vi "FPGA_Target_USB_7855R.vi"() -> ()   [LabVIEW 2023]
uses:
  <vilib>/eio/EIONode/EIONode.xnode
  <vilib>/rvi/eio/common/nirviEmuTemplateMethod_errors.vi
  <vilib>/rvi/DataTransferAndStorage/Container/XNode/niFpgaContainer.xnode
  <vilib>/rvi/interface/RandomDataEmulation/nirviRandomDataFpgaReadWriteTemplate.vi
  Tick Count.vi
  <vilib>/rvi/Memory/Memory_Emulation/nirvimemoryEmulation.vi
  <vilib>/rvi/Memory/Memory_Emulation/nirvimemoryFastEmulation.vi
  <vilib>/Platform/TimedLoop/XDataNode/wakeup.ctl
  <vilib>/Platform/TimedLoop/XDataNode/XDNodeRunTimeDep.lvlib
  <vilib>/Platform/TimedLoop/XDataNode/nitl_modes.ctl
  <vilib>/Platform/TimedLoop/XDataNode/timing_clust.ctl
  <vilib>/Platform/TimedLoop/XDataNode/XDataNode.xnode
  <vilib>/rvi/Arithmetic/AddSubMult/XNode/nirviSatArithmetic.xnode
  <vilib>/eio/EIOPropertyNode/EIOPropertyNode.xnode
  <vilib>/rvi/eio/common/nirviEmuTemplatePropertyGet_errors.vi
  <vilib>/rvi/eio/common/nirviEmuTemplatePropertyGet_noerrors.vi
  <vilib>/rvi/eio/common/nirviEmuTemplatePropertySet_errors.vi
  <vilib>/rvi/eio/common/nirviEmuTemplatePropertySet_noerrors.vi
panel:
  out "DIO0":bool
  out "CurrentMeasuredZ":i16
  out "CurrentMeasuredY":i16
  out "CalCoefAo0":cluster{"LSB Weight":u32, "Offset":i32}
  out "CalCoefAo1":cluster{"LSB Weight":u32, "Offset":i32}
  out "CalCoefAo2":cluster{"LSB Weight":u32, "Offset":i32}
  out "CalCoefAo3":cluster{"LSB Weight":u32, "Offset":i32}
  out "CalCoefAo4":cluster{"LSB Weight":u32, "Offset":i32}
  out "CalCoefAo5":cluster{"LSB Weight":u32, "Offset":i32}
  out "CalCoefAo6":cluster{"LSB Weight":u32, "Offset":i32}
  out "CalCoefAo7":cluster{"LSB Weight":u32, "Offset":i32}
  out "CalConstants Ready":bool
  out "CalCoefAi0":cluster{"LSB Weight":u32, "Offset":i32}
  out "CalCoefAi1":cluster{"LSB Weight":u32, "Offset":i32}
  out "CalCoefAi2":cluster{"LSB Weight":u32, "Offset":i32}
  out "CalCoefAi3":cluster{"LSB Weight":u32, "Offset":i32}
  out "CalCoefAi4":cluster{"LSB Weight":u32, "Offset":i32}
  out "CalCoefAi5":cluster{"LSB Weight":u32, "Offset":i32}
  out "CalCoefAi6":cluster{"LSB Weight":u32, "Offset":i32}
  out "CalCoefAi7":cluster{"LSB Weight":u32, "Offset":i32}
  out "Invert AO4 Output (V2)":bool
  out "Invert AO3 Output (V1)":bool
  out "Move Z Picomotor Direction":bool
  out "Move Z Picomotor":bool
  out "Tick Count(Ticks)":u32
  in  "HoldTimerScale":u64=18446744073709526080
  in  "Feedback1 on  Hold":bool
  out "Feedback2 Error":i32
  out "Feedback1 Error":i32
  out "Feedback2 Boolean":bool
  out "Feedback1 Boolean":bool
  out "ExtraTime 4":fxp<+,64,64>
  in  "DistanceToBulk 3":i16
  in  "DistanceToBulk 2":i16
  out "HasHeldHoldTimeHappend?":bool
  out "Z_axis_-10Vto10V":bool
  out "TraceRetraceFirstUse":bool
  in  "DistanceToBulk":i16
  out "V START":i16
  out "V END":i16
  out "X START":i16
  out "Y START":i16
  out "Z START":i16
  out "X END":i16
  out "Y END":i16
  out "Z END":i16
  out "V2 START":i16
  out "Count Average":i16
  out "AverageSum":i64
  out "IterateHolder":i16
  out "V2 VEl":i16
  out "V2 END":i16
  out "Update Position Loop Wait Time (ms)":u16=1
  out "LineType":i16
  out "V VEl":i16
  out "Z VEL":i16
  out "Y VEL":i16
  out "X VEL":i16
  out "Element":i16
  in  "V on Fly":i16=-32768
  in  "Change V on Fly":bool
  in  "Feedback_Threshold":i32
  in  "FeedBackType":u8
  out "x < y?":bool
  out "ExtraTime 3":fxp<+,64,64>
  in  "P2AvgMinus":i32
  out "ExtraTime 2":fxp<+,64,64>
  in  "P2AvgWhole":i32
  in  "Xoffset":u32
  in  "P":fxp<+/-,32,1>
  in  "Upper limit Of dZ":i32
  in  "FeedBackType 2":u8
  in  "Feedback_Threshold 2":i32
  in  "GreaterThan 2":bool
  in  "GreaterThan":bool
  in  "V2 on Fly":i16=-32768
  in  "Change V on Fly 2":bool
  out "CurrentMeasuredX":i16
  in  "2^(-n)":i16
  out "SampleNum":i16
  in  "Buffer Loop Wait Time (tICKS)":u32=1
  out "SampleIterator":i16
  out "Internal Stop":bool caption="Stop"
  out "MeasuredCurrent":i16=32767
  out "Applied Voltage":i16=-32768
  in  "External Stop":bool caption="Stop"
  in  "External Pause":bool
  out "Applied Z":i16
  out "Applied Y":i16
  out "Applied X":i16
  in  "Internal Pause":bool
  out "Accum Z":i32
  out "Accum I":i32
  out "Accum dV":i32
  out "Accum I2":i32
  out "OnlyStopLineONCE X":bool
  out "Accum Ext ac":i32
  out "Ext amp":i16=32767
  out "Accum Ext phase":i32
  in  "ExpandVelScaller X":i16=-27
  out "LineNumber":u64
  out "WaitingForWayPoints":bool caption="Stop"
  out "HoldTimer (ticks)":u64
  out "MeasuredCurrent 2":i16=32767
  out "Ext Phase":i16=32767
  in  "ExpandVelScaller Y":i16=-27
  in  "ExpandVelScaller Z":i16=-27
  in  "ExpandVelScaller V":i16=-27
  out "Accum I3":i32
  out "MeasuredCurrent 3":i16=32767
  out "MeasuredCurrent 4":i16=32767
  out "Accum Y":i32
  out "Accum X":i32
  out "OnlyStopLineONCE Y":bool
  out "OnlyStopLineONCE Z":bool
  out "OnlyStopLineONCE V":bool
  in  "EndCurrentLine":bool
  out "StopMoveX":bool
  out "StopMoveY":bool
  out "StopMoveZ":bool
  out "StopMoveV":bool
  out "Jump V":bool
  out "Stop Hold Position":bool
  out "Applied Voltage 2":i16
  out "StopMoveV2":bool
  out "Accum dV2":i32
  out "Jump V2":bool
  in  "ExpandVelScaller V2":i16=-27
  out "OnlyStopLineONCE V2":bool
  out "MoveAverage":i16
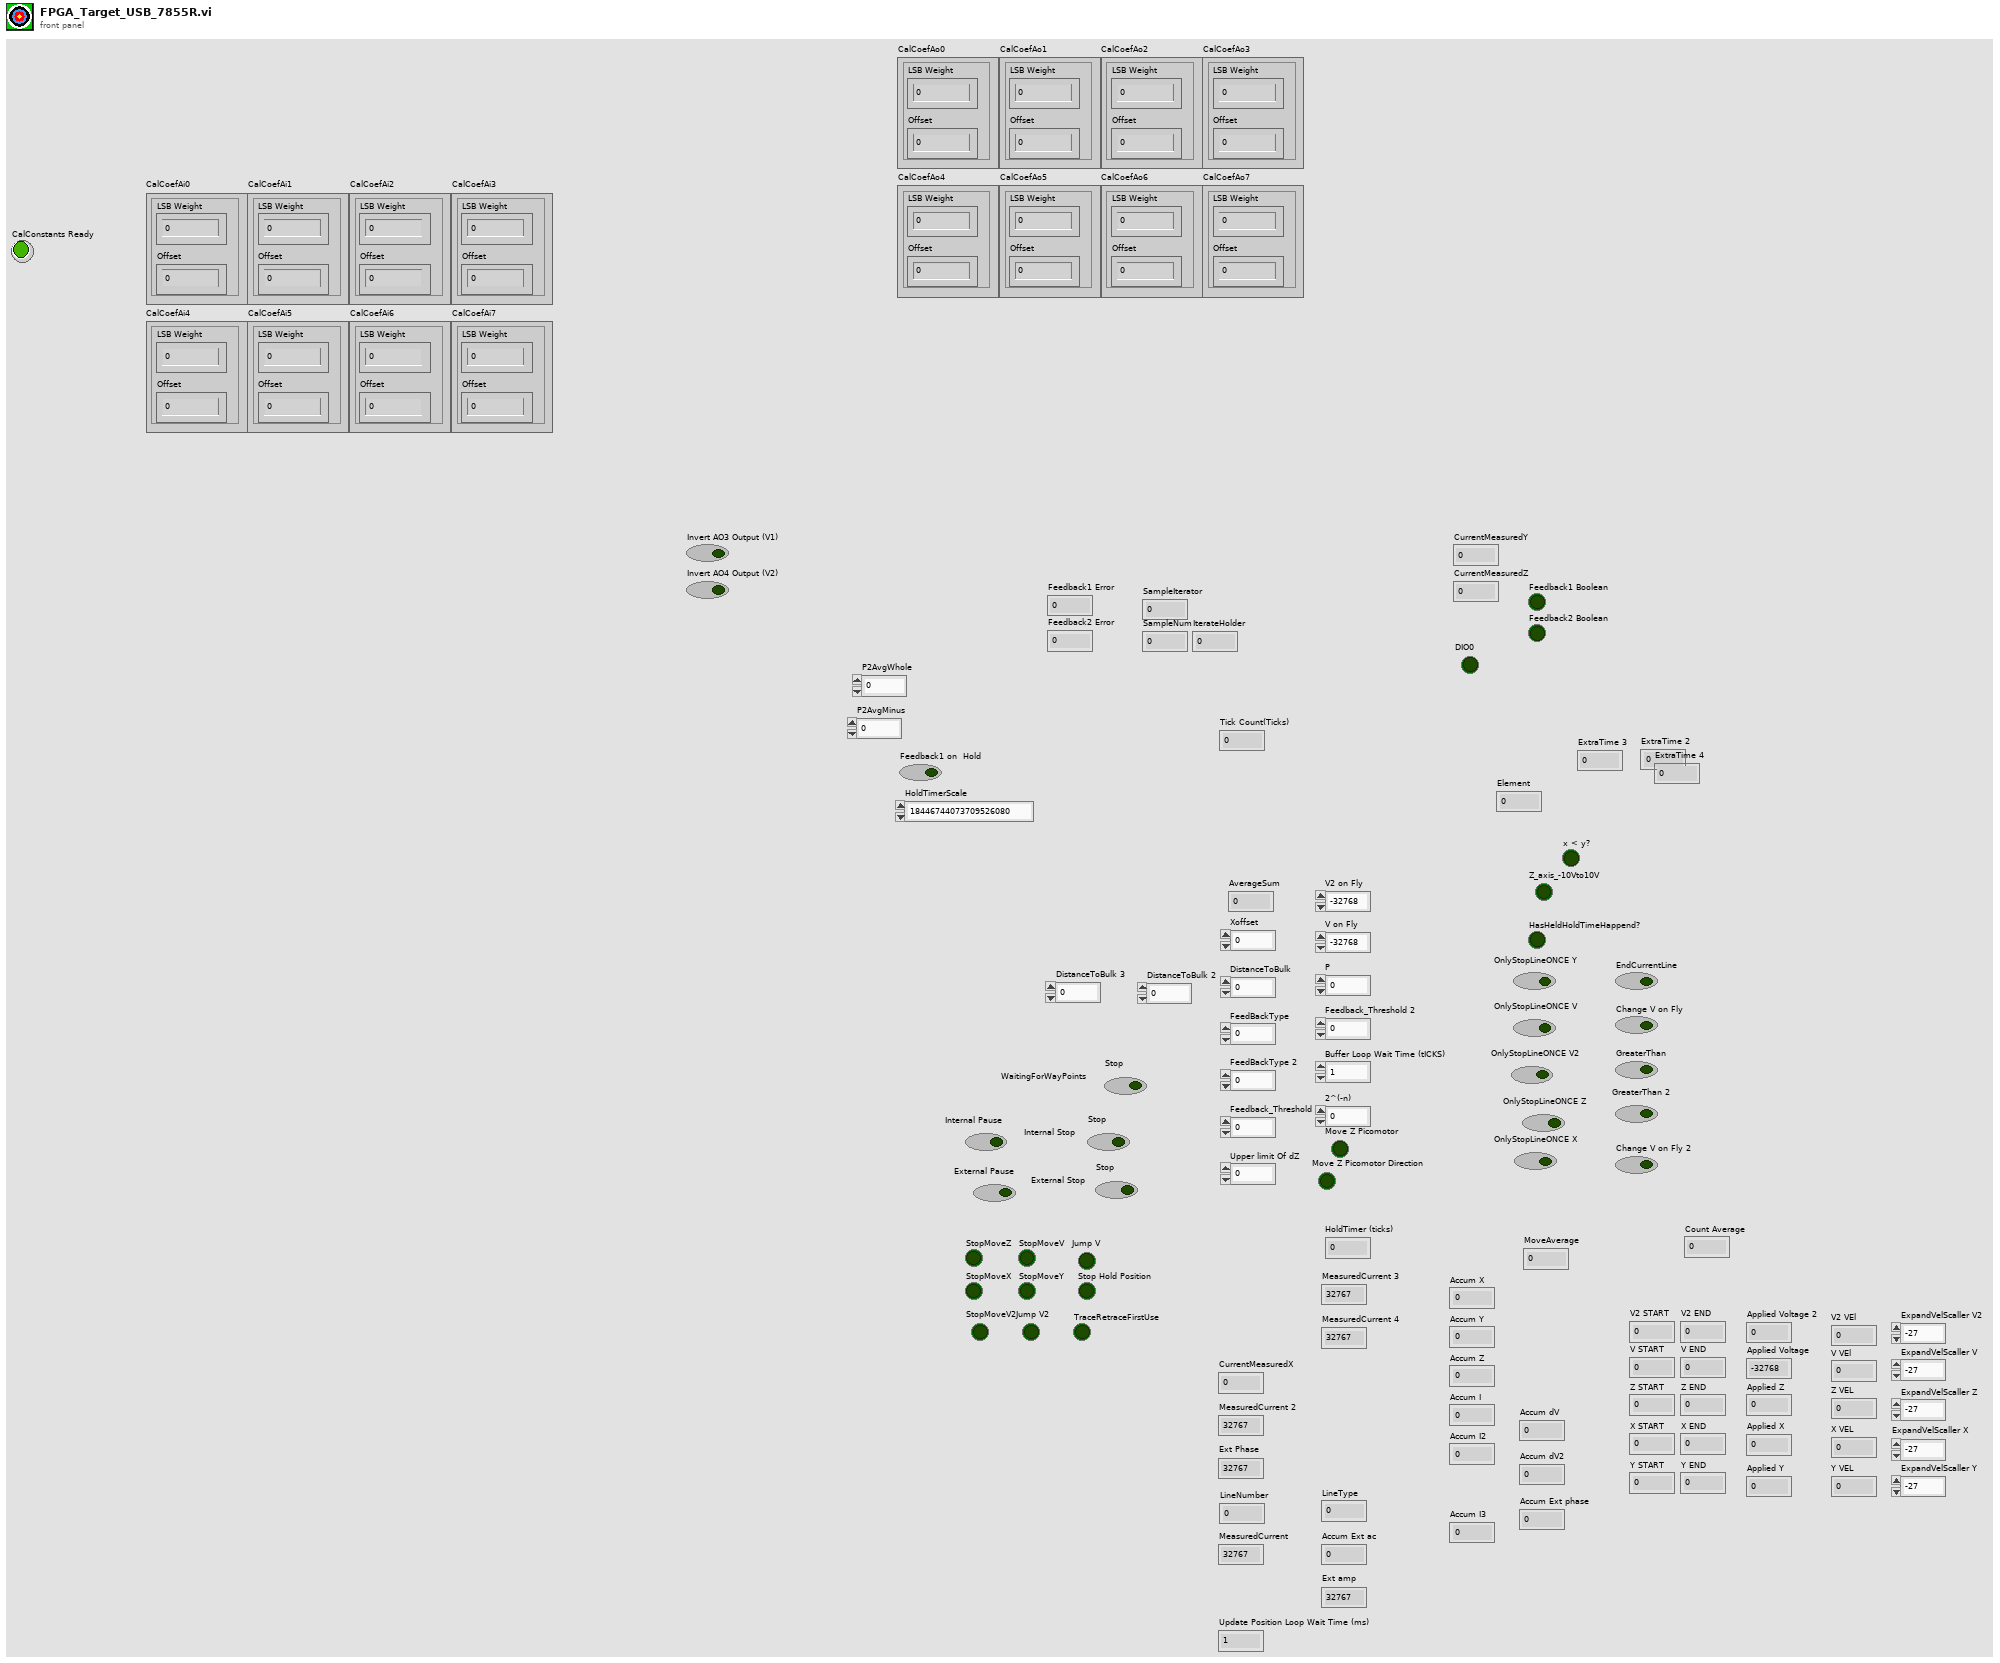
[diagram p1: front panel]
types:
  T1 = typedef "XDNodeRunTimeDep.lvlib/timing_clust.ctl" = cluster{"Expected End [f-1]":u64, "Actual End [f-1]":u64, "Finished Late? [f-1]":bool, "Expected End [i-1]":u64, "Actual End [i-1]":u64, "Finished Late? [i-1]":bool, "Expected Start [i]":u64, "Actual Start [i]":u64, "Expected Start [f]":u64, "Actual Start [f]":u64, "Source Name":string, "Structure Name":string, "Period":i64, "Deadline":i64, "Offset":i64, "Start":i64, "Priority":i32, "Timeout":i32, "Mode":T2, "Wakeup Reason":T3, "Error":errorcluster, "Source Type":string, "Secondary Source Type":string, "Global End Time":u64, "Global Start Time":u64, "Frame Duration":u64, "Iteration Duration":u64, "Assigned CPU":i32, "I/O Scan Engine Mode":u32}
  T2 = typedef "XDNodeRunTimeDep.lvlib/nitl_modes.ctl" = enum32{"No Change", "Process missed periods, maintain original phase", "Discard missed periods, maintain original phase", "Process missed periods, ignore original phase", "Discard missed periods, ignore original phase"}
  T3 = typedef "XDNodeRunTimeDep.lvlib/wakeup.ctl" = enum32{"Normal", "Aborted", "Asynchronous wakeup", "Timing source error", "Timed loop error", "Timeout"}
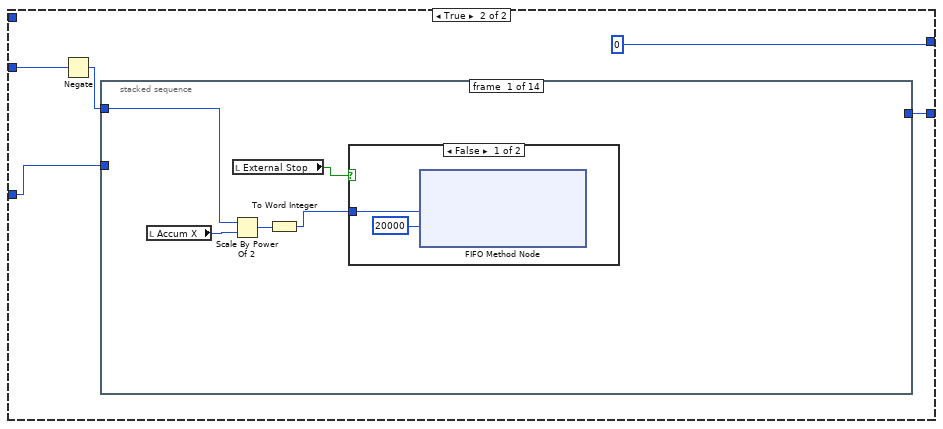
[diagram p2: hidden frame]
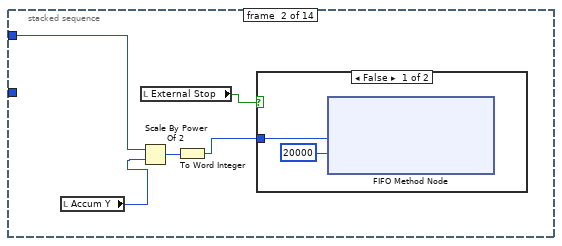
[diagram p4: hidden frame]
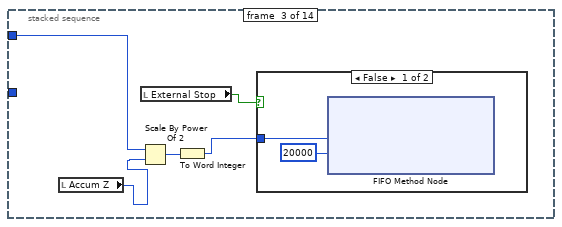
[diagram p6: hidden frame]
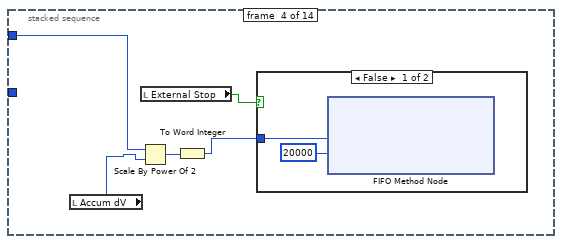
[diagram p8: hidden frame]
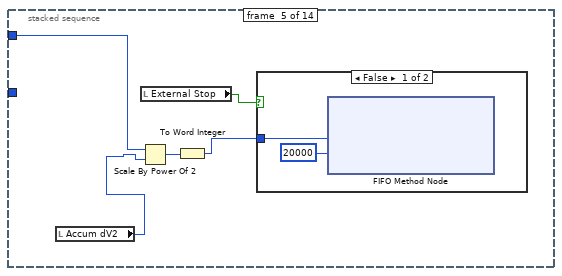
[diagram p10: hidden frame]
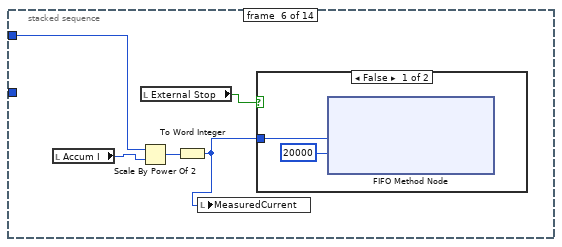
[diagram p12: hidden frame]
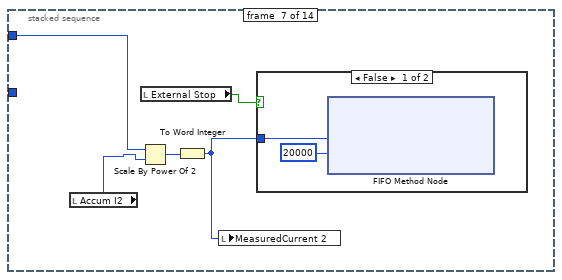
[diagram p14: hidden frame]
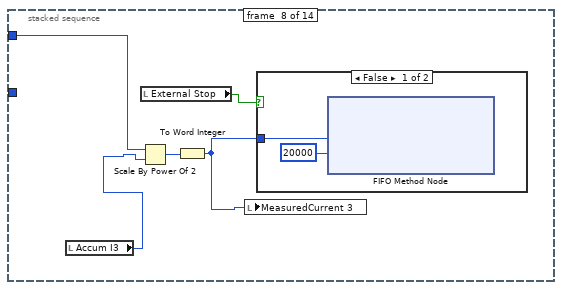
[diagram p16: hidden frame]
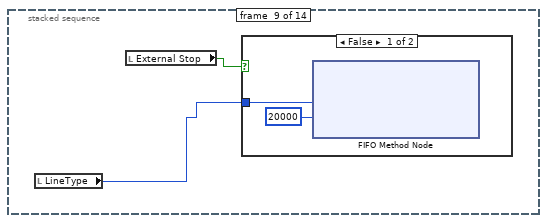
[diagram p18: hidden frame]
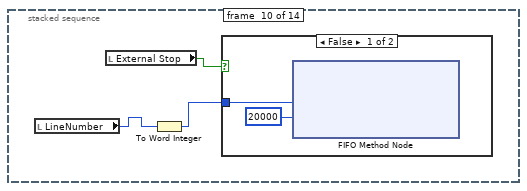
[diagram p20: hidden frame]
diagram:
  # "Increments  tick count by one every cycle, looping back to zero at ~2e19 ticks"
  n1 = node-c288() -> (w3:T1)  [unwired: 1 in]
  n2 = flat-sequence {
    frame #0 {
      w5 = FALSE ("Invert AO4 Output (V2)")
      w10 = FALSE ("OnlyStopLineONCE V2")
      w11 = FALSE ("Internal Stop")
      w4 = FALSE ("Internal Stop")
      w8 = u64 0 ("LineNumber")
      w7 = i16 0 ("Ext amp")
      w9 = i16 0 ("Applied Volatge")
      w18 = i16 32767 ("dZ Position")
      # "Set initial values of FP items and voltages to AO channels"
      "Internal Stop" <- FALSE ("Internal Stop")
      "MeasuredCurrent" <- w18
      "Applied Voltage" <- w9
      "Applied Z" <- i16 16383 ("Applied Volatge")
      "Applied Y" <- i16 16383 ("Applied Volatge")
      "Applied X" <- i16 16383 ("Applied Volatge")
      "Accum Z" <- 0 ("Applied Volatge")
      "Accum I" <- 0 ("Applied Volatge")
      "Accum dV" <- 0 ("Applied Volatge")
      "Accum I2" <- 0 ("Applied Volatge")
      "OnlyStopLineONCE X" <- w10
      "Accum Ext ac" <- 0 ("Accum Ext ac")
      "Ext amp" <- w7
      "Accum Ext phase" <- 0 ("Accum Ext phase")
      "LineNumber" <- w8
      "WaitingForWayPoints" <- FALSE ("WaitingForWayPoints")
      "HoldTimer (ticks)" <- w8
      "MeasuredCurrent 2" <- w18
      "Ext Phase" <- w7
      "Accum I3" <- 0 ("Applied Volatge")
      "MeasuredCurrent 3" <- w18
      "MeasuredCurrent 4" <- w18
      "Accum Y" <- 0 ("Applied Volatge")
      "Accum X" <- 0 ("Applied Volatge")
      "OnlyStopLineONCE Y" <- w10
      "OnlyStopLineONCE Z" <- w10
      "OnlyStopLineONCE V" <- w10
      "StopMoveX" <- w11
      "StopMoveY" <- w11
      "StopMoveZ" <- w11
      "StopMoveV" <- w11
      "Jump V" <- w4
      "Stop Hold Position" <- w4
      "Applied Voltage 2" <- w9
      "StopMoveV2" <- w11
      "Accum dV2" <- 0 ("Applied Volatge")
      "Jump V2" <- w4
      "OnlyStopLineONCE V2" <- w10
      "MoveAverage" <- w7
      "Z_axis_-10Vto10V" <- FALSE ("Internal Stop")
      "Move Z Picomotor" <- w4
      "Move Z Picomotor Direction" <- w4
      "Invert AO3 Output (V1)" <- w5
      "Invert AO4 Output (V2)" <- w5
      "DIO0" <- w4
    }
    frame #1 {
      w29 = i16 0  # SampleIterator
      n3 = while "Data Collection and Buffering Loop" {
        shift-right: [w34] -> _
        shift-left: w29 -> [w35]
        shift-right: [w32] -> _
        shift-left: u32 0 ("Tick Count(Ticks)") -> [w30]
        stop <- FALSE stop-if-true
        n4 = flat-sequence {
          tunnel: [w39] -> w36
          tunnel: w35 -> [w39]
          tunnel: w30 -> [w37]
          tunnel: [w37] -> w31
          tunnel: w36 -> [w47]
          tunnel: [w46] -> w34
          tunnel: [w41] -> w32
          tunnel: w31 -> [w40]
          frame #0 {
            n5 = call "Loop Timer2"("Count(Ticks)"="Buffer Loop Wait Time (tICKS)") -> ()  [unwired: 1 out]
          }
          frame #1 {
            n6 = Scale By Power Of 2(n="2^(-n)", x=i16 1) -> (x*2^n=w44:i16)
            "SampleNum" <- w44
            n7 = Greater Or Equal?(x=w47, y=w44) -> (x >= y?=w42:bool)
            n8 = case shown="False" w42 {
              tunnel: w47 -> [w90 _]
              tunnel: [w89 i16 0 ("lo")] -> w46
              tunnel: "2^(-n)" -> [_ w94]
              tunnel: [w48 w92] -> w41
              tunnel: w40 -> [w48 w91]
              frame False {
                n9 = xnode "FPGA I/O Node"() -> ("Connector1/AI0"=w53, "Connector1/AI1"=w60, "Connector1/AI2"=w77, "Connector1/AI3"=w76, "Connector1/AI4"=w75, "Connector1/AI5"=w74, "Connector1/AI6"=w67, "Connector1/AI7"=w64)  [unwired: 8 in, 8 out]
                "CurrentMeasuredX" <- w53
                "CurrentMeasuredY" <- w60
                "CurrentMeasuredZ" <- w77
                n10 = local read "Applied Voltage 2"() -> (w51:i16)
                n11 = local read "Applied Voltage"() -> (w79:i16)
                n12 = Increment(x=w90) -> (x+1=w89:i16)
                n13 = To Long Integer(number=w79) -> (32bit integer=w78:i32)
                n14 = To Long Integer(number=w51) -> (32bit integer=w52:i32)
                n15 = To Long Integer(number=w64) -> (32bit integer=w63:i32)
                n16 = To Long Integer(number=w77) -> (32bit integer=w61:i32)
                n17 = To Long Integer(number=w53) -> (32bit integer=w54:i32)
                n18 = To Long Integer(number=w60) -> (32bit integer=w59:i32)
                n19 = To Long Integer(number=w74) -> (32bit integer=w73:i32)
                n20 = local read "Accum dV2"() -> (w49:i32)
                n21 = local read "Accum dV"() -> (w81:i32)
                n22 = To Long Integer(number=w75) -> (32bit integer=w83:i32)
                n23 = local read "Accum I3"() -> (w65:i32)
                n24 = To Long Integer(number=w76) -> (32bit integer=w86:i32)
                n25 = local read "Accum X"() -> (w55:i32)
                n26 = local read "Accum Ext phase"() -> (w69:i32)
                n27 = local read "Accum Y"() -> (w58:i32)
                n28 = local read "Accum I2"() -> (w84:i32)
                n29 = local read "Accum Ext ac"() -> (w72:i32)
                n30 = local read "Accum Z"() -> (w62:i32)
                n31 = local read "Accum I"() -> (w87:i32)
                n32 = Add(x=w81, y=w78) -> (x+y=w80:i32)
                n33 = Add(x=w49, y=w52) -> (x+y=w50:i32)
                n34 = To Long Integer(number=w67) -> (32bit integer=w68:i32)
                n35 = Add(x=w55, y=w54) -> (x+y=w56:i32)
                n36 = Add(x=w58, y=w59) -> (x+y=w57:i32)
                n37 = Add(x=w62, y=w61) -> (x+y=w88:i32)
                n38 = Add(x=w84, y=w83) -> (x+y=w82:i32)
                n39 = Add(x=w63, y=w65) -> (x+y=w66:i32)
                n40 = Add(x=w87, y=w86) -> (x+y=w85:i32)
                n41 = Add(x=w68, y=w69) -> (x+y=w70:i32)
                n42 = Add(x=w72, y=w73) -> (x+y=w71:i32)
                n43 = local write "Accum dV2"(w50) -> ()
                n44 = local write "Accum dV"(w80) -> ()
                n45 = local write "Accum X"(w56) -> ()
                n46 = local write "Accum Ext phase"(w70) -> ()
                n47 = local write "Accum Y"(w57) -> ()
                n48 = local write "Accum Ext ac"(w71) -> ()
                n49 = local write "Accum Z"(w88) -> ()
                n50 = local write "Accum I2"(w82) -> ()
                n51 = local write "Accum I"(w85) -> ()
                n52 = local write "Accum I3"(w66) -> ()
              }
              frame True {
                n53 = Negate(x=w94) -> (-x=w93:i16)
                n54 = stacked-sequence {
                  tunnel: w93 -> [w96 w104 w111 w119 w126 w133 w140 w147 _ _ w164 w171 _ _]
                  tunnel: [_ _ _ _ _ _ _ _ _ _ _ _ w177 _] -> w92
                  tunnel: w91 -> [_ _ _ _ _ _ _ _ _ _ _ _ w176 _]
                  frame #0 {
                    n55 = local read "Accum X"() -> (w97:i32)
                    n56 = Scale By Power Of 2(n=w96, x=w97) -> (x*2^n=w98:i32)
                    n57 = local read "External Stop"() -> (w99:bool)
                    n58 = To Word Integer(number=w98) -> (16bit integer=w100:i16)
                    n59 = case shown="False" w99 {
                      tunnel: w100 -> [w101 _]
                      frame False {
                        n60 = xnode ("FIFO Method Node")("Element"=w101, "Timeout"=20000) -> ()  [unwired: 1 in, 2 out]
                      }
                      frame True {
                      }
                    }
                  }
                  frame #1 {
                    n61 = local read "Accum Y"() -> (w103:i32)
                    n62 = Scale By Power Of 2(n=w104, x=w103) -> (x*2^n=w105:i32)
                    n63 = local read "External Stop"() -> (w106:bool)
                    n64 = To Word Integer(number=w105) -> (16bit integer=w107:i16)
                    n65 = case shown="False" w106 {
                      tunnel: w107 -> [w108 _]
                      frame False {
                        n66 = xnode ("FIFO Method Node")("Element"=w108, "Timeout"=20000) -> ()  [unwired: 1 in, 2 out]
                      }
                      frame True {
                      }
                    }
                  }
                  frame #2 {
                    n67 = local read "Accum Z"() -> (w110:i32)
                    n68 = Scale By Power Of 2(n=w111, x=w110) -> (x*2^n=w112:i32)
                    n69 = local read "External Stop"() -> (w113:bool)
                    n70 = To Word Integer(number=w112) -> (16bit integer=w114:i16)
                    n71 = case shown="False" w113 {
                      tunnel: w114 -> [w115 _]
                      frame False {
                        n72 = xnode ("FIFO Method Node")("Element"=w115, "Timeout"=20000) -> ()  [unwired: 1 in, 2 out]
                      }
                      frame True {
                      }
                    }
                  }
                  frame #3 {
                    n73 = local read "Accum dV"() -> (w117:i32)
                    n74 = Scale By Power Of 2(n=w119, x=w117) -> (x*2^n=w120:i32)
                    n75 = local read "External Stop"() -> (w121:bool)
                    n76 = To Word Integer(number=w120) -> (16bit integer=w118:i16)
                    n77 = case shown="False" w121 {
                      tunnel: w118 -> [w122 _]
                      frame False {
                        n78 = xnode ("FIFO Method Node")("Element"=w122, "Timeout"=20000) -> ()  [unwired: 1 in, 2 out]
                      }
                      frame True {
                      }
                    }
                  }
                  frame #4 {
                    n79 = local read "Accum dV2"() -> (w124:i32)
                    n80 = Scale By Power Of 2(n=w126, x=w124) -> (x*2^n=w127:i32)
                    n81 = local read "External Stop"() -> (w128:bool)
                    n82 = To Word Integer(number=w127) -> (16bit integer=w125:i16)
                    n83 = case shown="False" w128 {
                      tunnel: w125 -> [w129 _]
                      frame False {
                        n84 = xnode ("FIFO Method Node")("Element"=w129, "Timeout"=20000) -> ()  [unwired: 1 in, 2 out]
                      }
                      frame True {
                      }
                    }
                  }
                  frame #5 {
                    n85 = local read "Accum I"() -> (w132:i32)
                    n86 = Scale By Power Of 2(n=w133, x=w132) -> (x*2^n=w134:i32)
                    n87 = local read "External Stop"() -> (w135:bool)
                    n88 = To Word Integer(number=w134) -> (16bit integer=w131:i16)
                    n89 = local write "MeasuredCurrent"(w131) -> ()
                    n90 = case shown="False" w135 {
                      tunnel: w131 -> [w136 _]
                      frame False {
                        n91 = xnode ("FIFO Method Node")("Element"=w136, "Timeout"=20000) -> ()  [unwired: 1 in, 2 out]
                      }
                      frame True {
                      }
                    }
                  }
                  frame #6 {
                    n92 = local read "Accum I2"() -> (w139:i32)
                    n93 = Scale By Power Of 2(n=w140, x=w139) -> (x*2^n=w141:i32)
                    n94 = local read "External Stop"() -> (w142:bool)
                    n95 = To Word Integer(number=w141) -> (16bit integer=w138:i16)
                    n96 = local write "MeasuredCurrent 2"(w138) -> ()
                    n97 = case shown="False" w142 {
                      tunnel: w138 -> [w143 _]
                      frame False {
                        n98 = xnode ("FIFO Method Node")("Element"=w143, "Timeout"=20000) -> ()  [unwired: 1 in, 2 out]
                      }
                      frame True {
                      }
                    }
                  }
                  frame #7 {
                    n99 = local read "Accum I3"() -> (w146:i32)
                    n100 = Scale By Power Of 2(n=w147, x=w146) -> (x*2^n=w148:i32)
                    n101 = local read "External Stop"() -> (w149:bool)
                    n102 = To Word Integer(number=w148) -> (16bit integer=w145:i16)
                    n103 = local write "MeasuredCurrent 3"(w145) -> ()
                    n104 = case shown="False" w149 {
                      tunnel: w145 -> [w150 _]
                      frame False {
                        n105 = xnode ("FIFO Method Node")("Element"=w150, "Timeout"=20000) -> ()  [unwired: 1 in, 2 out]
                      }
                      frame True {
                      }
                    }
                  }
                  frame #8 {
                    n106 = local read "LineType"() -> (w152:i16)
                    n107 = local read "External Stop"() -> (w153:bool)
                    n108 = case shown="False" w153 {
                      tunnel: w152 -> [w154 _]
                      frame False {
                        n109 = xnode ("FIFO Method Node")("Element"=w154, "Timeout"=20000) -> ()  [unwired: 1 in, 2 out]
                      }
                      frame True {
                      }
                    }
                  }
                  frame #9 {
                    n110 = local read "LineNumber"() -> (w157:u64)
                    n111 = local read "External Stop"() -> (w158:bool)
                    n112 = To Word Integer(number=w157) -> (16bit integer=w156:i16)
                    n113 = case shown="False" w158 {
                      tunnel: w156 -> [w159 _]
                      frame False {
                        n114 = xnode ("FIFO Method Node")("Element"=w159, "Timeout"=20000) -> ()  [unwired: 1 in, 2 out]
                      }
                      frame True {
                      }
                    }
                  }
                  frame #10 {
                    n115 = local read "Accum Ext ac"() -> (w163:i32)
                    n116 = local read "External Stop"() -> (w165:bool)
                    n117 = Scale By Power Of 2(n=w164, x=w163) -> (x*2^n=w162:i32)
                    n118 = To Word Integer(number=w162) -> (16bit integer=w161:i16)
                    n119 = case shown="False" w165 {
                      tunnel: w161 -> [w166 _]
                      frame False {
                        n120 = xnode ("FIFO Method Node")("Element"=w166, "Timeout"=20000) -> ()  [unwired: 1 in, 2 out]
                      }
                      frame True {
                      }
                    }
                    n121 = local write "Ext amp"(w161) -> ()
                  }
                  frame #11 {
                    n122 = local read "Accum Ext phase"() -> (w169:i32)
                    n123 = local read "External Stop"() -> (w172:bool)
                    n124 = Scale By Power Of 2(n=w171, x=w169) -> (x*2^n=w170:i32)
                    n125 = To Word Integer(number=w170) -> (16bit integer=w168:i16)
                    n126 = local write "Ext Phase"(w168) -> ()
                    n127 = case shown="False" w172 {
                      tunnel: w168 -> [w173 _]
                      frame False {
                        n128 = xnode ("FIFO Method Node")("Element"=w173, "Timeout"=20000) -> ()  [unwired: 1 in, 2 out]
                      }
                      frame True {
                      }
                    }
                  }
                  frame #12 {
                    n129 = call "Tick Count"() -> ("Tick Count(Ticks)"=w177:u32)
                    n130 = Subtract(x=w177, y=w176) -> (x-y=w175:u32)
                    "Tick Count(Ticks)" <- w175
                    n131 = local read "External Stop"() -> (w188:bool)
                    n132 = Split Number(x=w175) -> (hi(x)=w187:u16, lo(x)=w179:u16)
                    n133 = To Long Integer(number=w179) -> (32bit integer=w180:i32)
                    n134 = To Long Integer(number=w187) -> (32bit integer=w186:i32)
                    n135 = Subtract(x=w180, y=32768) -> (x-y=w182:i32)
                    n136 = Subtract(x=w186, y=32768) -> (x-y=w184:i32)
                    n137 = To Word Integer(number=w182) -> (16bit integer=w178:i16)
                    n138 = To Word Integer(number=w184) -> (16bit integer=w183:i16)
                    n139 = case shown="False" w188 {
                      tunnel: w183 -> [w190 _]
                      tunnel: w178 -> [w189 _]
                      frame False {
                        n140 = flat-sequence {
                          tunnel: w190 -> [w191]
                          tunnel: w189 -> [w193]
                          frame #0 {
                            n141 = xnode ("FIFO Method Node")("Element"=w191, "Timeout"=20000) -> ()  [unwired: 1 in, 2 out]
                          }
                          frame #1 {
                            n142 = xnode ("FIFO Method Node")("Element"=w193, "Timeout"=20000) -> ()  [unwired: 1 in, 2 out]
                          }
                        }
                      }
                      frame True {
                      }
                    }
                  }
                  frame #13 {
                    n143 = local write "Accum dV"(0 ("MeasuredCurrent")) -> ()
                    n144 = local write "Accum Z"(0 ("MeasuredCurrent")) -> ()
                    n145 = local write "Accum dV2"(0 ("Accum Ext ac")) -> ()
                    n146 = local write "Accum I2"(0 ("MeasuredCurrent")) -> ()
                    n147 = local write "Accum I"(0 ("MeasuredCurrent")) -> ()
                    n148 = local write "Accum Y"(0 ("Accum Ext ac")) -> ()
                    n149 = local write "Accum X"(0 ("MeasuredCurrent")) -> ()
                    n150 = local write "Accum Ext ac"(0 ("Accum Ext ac")) -> ()
                    n151 = local write "Accum I3"(0 ("Accum Ext ac")) -> ()
                    n152 = local write "Accum Ext phase"(0 ("Accum Ext phase")) -> ()
                  }
                }
              }
            }
          }
        }
        "SampleIterator" <- w35
      }
      n153 = while "X Y Z Voltage" {
        stop <- FALSE stop-if-true
        # "Load Waypoints"
        n154 = flat-sequence {
          tunnel: [w1129] -> w206
          tunnel: [w1128] -> w212
          tunnel: [w1127] -> w211
          tunnel: [w1126] -> w210
          tunnel: [w1125] -> w209
          tunnel: [w1124] -> w208
          tunnel: [w1122] -> w207
          tunnel: [w1121] -> w205
          frame #0 {
            n155 = while {
              shift-right: [w922] -> _
              shift-left: TRUE ("WaitingForWayPoints") -> [w923]
              stop <- w926 stop-if-true
              n156 = xnode ("FIFO Method Node")() -> ("Number of Elements to Read"=w931:u32)  [unwired: 1 in, 1 out]
              n157 = local read "External Stop"() -> (w924:bool)
              n158 = And(x=w924, y=w923) -> (x .and. y?=w925:bool)
              n159 = case shown="True" w925 {
                tunnel: w923 -> [w932 _]
                tunnel: [w932 FALSE ("WaitingForWayPoints")] -> w922
                frame False {
                }
                frame True {
                  n160 = while {
                    stop <- w934 stop-if-true
                    n161 = xnode ("FIFO Method Node")("Timeout"=100) -> ("Element"=→"Element":i16, "Timed Out?"=w934:bool)  [unwired: 1 in, 1 out]
                  }
                }
              }
              n162 = Greater?(x=w931, y=u32 13) -> (0:w927:bool)
              n163 = Not(x=w927) -> (.not. x?=w929:bool)
              n164 = local write "WaitingForWayPoints"(w929) -> ()
              n165 = Not(x=w924) -> (.not. x?=w928:bool)
              n166 = And(x=w928, y=w927) -> (x .and. y?=w926:bool)
            }
          }
          frame #1 {
            n167 = stacked-sequence {
              frame #0 {
                n168 = xnode ("FIFO Method Node")("Timeout"=-1) -> ("Element"=→"LineType":i16)  [unwired: 1 in, 2 out]
              }
              frame #1 {
                n169 = xnode ("FIFO Method Node")("Timeout"=-1) -> ("Element"=→"X VEL":i16)  [unwired: 1 in, 2 out]
              }
              frame #2 {
                n170 = xnode ("FIFO Method Node")("Timeout"=-1) -> ("Element"=→"Y VEL":i16)  [unwired: 1 in, 2 out]
              }
              frame #3 {
                n171 = xnode ("FIFO Method Node")("Timeout"=-1) -> ("Element"=→"Z VEL":i16)  [unwired: 1 in, 2 out]
              }
              frame #4 {
                n172 = xnode ("FIFO Method Node")("Timeout"=-1) -> ("Element"=→"V VEl":i16)  [unwired: 1 in, 2 out]
              }
              frame #5 {
                n173 = xnode ("FIFO Method Node")("Timeout"=-1) -> ("Element"=→"V2 VEl":i16)  [unwired: 1 in, 2 out]
              }
              frame #6 {
                n174 = xnode ("FIFO Method Node")("Timeout"=-1) -> ("Element"=→"X END":i16)  [unwired: 1 in, 2 out]
              }
              frame #7 {
                n175 = xnode ("FIFO Method Node")("Timeout"=-1) -> ("Element"=→"Y END":i16)  [unwired: 1 in, 2 out]
              }
              frame #8 {
                n176 = xnode ("FIFO Method Node")("Timeout"=-1) -> ("Element"=w954:i16)  [unwired: 1 in, 2 out]
                n177 = local read "LineType"() -> (w955:i16)
                n178 = case shown="13" w955 {
                  tunnel: [w957 w962 w974 w986 w994] -> w953
                  tunnel: w954 -> [w957 _ _ _ _]
                  frame 0..2, Default {
                    # "Normal Move"
                  }
                  frame 3 {
                    # "Bulk At End Of line - Retract"
                    n179 = local read "Z_axis_-10Vto10V"() -> (w961:bool)
                    n180 = local read "Applied Z"() -> (w969:i16)
                    n181 = Select(t=-32768 ("lower limit"), s=w961, f=0 ("lower limit")) -> (s? t:f=w960:i32)
                    n182 = To Long Integer(number=w969) -> (32bit integer=w966:i32)
                    n183 = To Long Integer(number="DistanceToBulk") -> (32bit integer=w967:i32)
                    n184 = Add(x=w966, y=w967) -> (x+y=w965:i32)
                    n185 = In Range and Coerce(upper limit=32767, x=w965, lower limit=w960) -> (coerced(x)=w963:i32)  [unwired: 1 out]
                    n186 = To Word Integer(number=w963) -> (16bit integer=w962:i16)
                  }
                  frame 12 {
                    # "Bulk At End Of line - Retract"
                    n187 = local read "Z_axis_-10Vto10V"() -> (w973:bool)
                    n188 = local read "Applied Z"() -> (w981:i16)
                    n189 = Select(t=-32768 ("lower limit"), s=w973, f=0 ("lower limit")) -> (s? t:f=w972:i32)
                    n190 = To Long Integer(number=w981) -> (32bit integer=w978:i32)
                    n191 = To Long Integer(number="DistanceToBulk 2") -> (32bit integer=w979:i32)
                    n192 = Add(x=w978, y=w979) -> (x+y=w977:i32)
                    n193 = In Range and Coerce(upper limit=32767, x=w977, lower limit=w972) -> (coerced(x)=w975:i32)  [unwired: 1 out]
                    n194 = To Word Integer(number=w975) -> (16bit integer=w974:i16)
                  }
                  frame 13 {
                    # "Bulk At End Of line - Retract"
                    n195 = local read "Z_axis_-10Vto10V"() -> (w985:bool)
                    n196 = local read "Applied Z"() -> (w993:i16)
                    n197 = Select(t=-32768 ("lower limit"), s=w985, f=0 ("lower limit")) -> (s? t:f=w984:i32)
                    n198 = To Long Integer(number=w993) -> (32bit integer=w990:i32)
                    n199 = To Long Integer(number="DistanceToBulk 3") -> (32bit integer=w991:i32)
                    n200 = Add(x=w990, y=w991) -> (x+y=w989:i32)
                    n201 = In Range and Coerce(upper limit=32767, x=w989, lower limit=w984) -> (coerced(x)=w987:i32)  [unwired: 1 out]
                    n202 = To Word Integer(number=w987) -> (16bit integer=w986:i16)
                  }
                  frame 4..7 {
                    # "Start at current hieght"
                    n203 = local read "Applied Z"() -> (w994:i16)
                  }
                }
                "Z END" <- w953
              }
              frame #9 {
                n204 = xnode ("FIFO Method Node")("Timeout"=-1) -> ("Element"=→"V END":i16)  [unwired: 1 in, 2 out]
              }
              frame #10 {
                n205 = xnode ("FIFO Method Node")("Timeout"=-1) -> ("Element"=→"V2 END":i16)  [unwired: 1 in, 2 out]
              }
              frame #11 {
                n206 = xnode ("FIFO Method Node")("Timeout"=-1) -> ("Element"=w1000:i16)  [unwired: 1 in, 2 out]
                n207 = To Unsigned Word Integer(number=w1000) -> (unsigned 16bit integer=→"Update Position Loop Wait Time (ms)":u16)
              }
              frame #12 {
                n208 = flat-sequence {
                  tunnel: [w1008] -> w1004
                  tunnel: [w1010] -> w1003
                  frame #0 {
                    n209 = xnode ("FIFO Method Node")("Timeout"=-1) -> ("Element"=w1008:i16)  [unwired: 1 in, 2 out]
                  }
                  frame #1 {
                    n210 = xnode ("FIFO Method Node")("Timeout"=-1) -> ("Element"=w1010:i16)  [unwired: 1 in, 2 out]
                  }
                }
                n211 = Join Numbers(hi=w1004, lo=w1003) -> ((hi.lo)=w1002:u32)
                n212 = To Unsigned Quad Integer(1:w1002) -> (0:w1007:u64)
                n213 = Multiply(x=w1007, y="HoldTimerScale") -> (x*y=w1005:u64)
                n214 = local write "HoldTimer (ticks)"(w1005) -> ()
              }
              frame #13 {
                n215 = xnode ("FIFO Method Node")("Timeout"=-1) -> ("Element"=w1023:i16)  [unwired: 1 in, 2 out]
                n216 = Number To Boolean Array(number=w1023) -> (Boolean array=w1013:bool[])
                n217 = Index Array(array=w1013, index=0) -> (element=w1028:bool)
                n218 = Index Array(array=w1013, index=1) -> (element=w1029:bool)
                n219 = Index Array(array=w1013, index=2) -> (element=w1033:bool)
                n220 = Index Array(array=w1013, index=4) -> (element=w1038:bool)
                n221 = Index Array(array=w1013, index=5) -> (element=w1022:bool)
                n222 = Index Array(array=w1013, index=3) -> (element=w1030:bool)
                n223 = Index Array(array=w1013, index=10) -> (element=w1016:bool)
                n224 = Index Array(array=w1013, index=9) -> (element=w1017:bool)
                n225 = Index Array(array=w1013, index=11) -> (element=w1012:bool)
                n226 = Index Array(array=w1013, index=6) -> (element=w1040:bool)
                n227 = Not(x=w1030) -> (.not. x?=w1037:bool)
                n228 = Not(x=w1028) -> (.not. x?=w1034:bool)
                n229 = Not(x=w1022) -> (.not. x?=w1021:bool)
                n230 = Index Array(array=w1013, index=7) -> (element=w1043:bool)
                n231 = Index Array(array=w1013, index=8) -> (element=w1019:bool)
                n232 = Not(x=w1033) -> (.not. x?=w1036:bool)
                n233 = Not(x=w1029) -> (.not. x?=w1035:bool)
                n234 = local write "StopMoveX"(w1034) -> ()
                n235 = local write "Stop Hold Position"(w1021) -> ()
                n236 = Not(x=w1040) -> (.not. x?=w1041:bool)
                n237 = local write "Move Z Picomotor Direction"(w1016) -> ()
                n238 = local write "StopMoveY"(w1035) -> ()
                n239 = local write "StopMoveZ"(w1036) -> ()
                n240 = local write "StopMoveV2"(w1041) -> ()
                n241 = local write "StopMoveV"(w1037) -> ()
                n242 = local write "DIO0"(w1012) -> ()
                n243 = local write "Move Z Picomotor"(w1017) -> ()
                n244 = local write "Jump V"(w1038) -> ()
                n245 = local write "Feedback1 on  Hold"(w1019) -> ()
                n246 = local write "Jump V2"(w1043) -> ()
              }
            }
          }
          frame #2 {
            # "Initial Positions, Always start at the current Position"
            n247 = local read "LineNumber"() -> (w1050:u64)
            n248 = local read "Applied Voltage"() -> (→"V START":i16)
            n249 = local read "Applied Voltage 2"() -> (→"V2 START":i16)
            n250 = local read "Applied Z"() -> (→"Z START":i16)
            n251 = local read "Applied X"() -> (→"X START":i16)
            n252 = local read "Applied Y"() -> (→"Y START":i16)
            n253 = local read "SampleNum"() -> (→"IterateHolder":i16)
            n254 = Increment(x=w1050) -> (x+1=w1049:u64)
            n255 = local write "LineNumber"(w1049) -> ()
            "Count Average" <- i16 0
            "AverageSum" <- i64 0 ("LineNumber")
          }
          frame #3 {
            # "Make Sure the Velocity is pointing in the right direction"
            n256 = local read "X START"() -> (w1069:i16)
            n257 = local read "Y START"() -> (w1064:i16)
            n258 = local read "V2 START"() -> (w1057:i16)
            n259 = local read "X END"() -> (w1068:i16)
            n260 = local read "V START"() -> (w1058:i16)
            n261 = local read "Z START"() -> (w1063:i16)
            n262 = local read "V2 END"() -> (w1056:i16)
            n263 = local read "V END"() -> (w1059:i16)
            n264 = local read "Y END"() -> (w1065:i16)
            n265 = local read "Z END"() -> (w1062:i16)
            n266 = Greater?(x=w1069, y=w1068) -> (0:w1067:bool)
            n267 = Greater?(x=w1064, y=w1065) -> (0:w1066:bool)
            n268 = Greater?(x=w1058, y=w1059) -> (0:w1060:bool)
            n269 = Greater?(x=w1063, y=w1062) -> (0:w1061:bool)
            n270 = Greater?(x=w1057, y=w1056) -> (0:w1055:bool)
            n271 = case shown="False" w1067 {
              frame False {
                n272 = local read "X VEL"() -> (w1110:i16)
                n273 = Greater?(x=w1110, y=i16 0) -> (0:w1111:bool)
                n274 = case shown="False" w1111 {
                  tunnel: w1110 -> [w1114 _]
                  frame False {
                    n275 = Negate(x=w1114) -> (-x=w1113:i16)
                    n276 = local write "X VEL"(w1113) -> ()
                  }
                  frame True {
                  }
                }
              }
              frame True {
                n277 = local read "X VEL"() -> (w1115:i16)
                n278 = Greater?(x=w1115, y=i16 0) -> (0:w1116:bool)
                n279 = case shown="True" w1116 {
                  tunnel: w1115 -> [_ w1119]
                  frame False {
                  }
                  frame True {
                    n280 = Negate(x=w1119) -> (-x=w1118:i16)
                    n281 = local write "X VEL"(w1118) -> ()
                  }
                }
              }
            }
            n282 = case shown="True" w1066 {
              frame False {
                n283 = local read "Y VEL"() -> (w1100:i16)
                n284 = Greater?(x=w1100, y=i16 0) -> (0:w1101:bool)
                n285 = case shown="False" w1101 {
                  tunnel: w1100 -> [w1104 _]
                  frame False {
                    n286 = Negate(x=w1104) -> (-x=w1103:i16)
                    n287 = local write "Y VEL"(w1103) -> ()
                  }
                  frame True {
                  }
                }
              }
              frame True {
                n288 = local read "Y VEL"() -> (w1105:i16)
                n289 = Greater?(x=w1105, y=i16 0) -> (0:w1106:bool)
                n290 = case shown="True" w1106 {
                  tunnel: w1105 -> [_ w1109]
                  frame False {
                  }
                  frame True {
                    n291 = Negate(x=w1109) -> (-x=w1108:i16)
                    n292 = local write "Y VEL"(w1108) -> ()
                  }
                }
              }
            }
            n293 = case shown="True" w1060 {
              frame False {
                n294 = local read "V VEl"() -> (w1080:i16)
                n295 = Greater?(x=w1080, y=i16 0) -> (0:w1081:bool)
                n296 = case shown="False" w1081 {
                  tunnel: w1080 -> [w1084 _]
                  frame False {
                    n297 = Negate(x=w1084) -> (-x=w1083:i16)
                    n298 = local write "V VEl"(w1083) -> ()
                  }
                  frame True {
                  }
                }
              }
              frame True {
                n299 = local read "V VEl"() -> (w1085:i16)
                n300 = Greater?(x=w1085, y=i16 0) -> (0:w1086:bool)
                n301 = case shown="True" w1086 {
                  tunnel: w1085 -> [_ w1089]
                  frame False {
                  }
                  frame True {
                    n302 = Negate(x=w1089) -> (-x=w1088:i16)
                    n303 = local write "V VEl"(w1088) -> ()
                  }
                }
              }
            }
            n304 = case shown="True" w1061 {
              frame False {
                n305 = local read "Z VEL"() -> (w1090:i16)
                n306 = Greater?(x=w1090, y=i16 0) -> (0:w1091:bool)
                n307 = case shown="False" w1091 {
                  tunnel: w1090 -> [w1094 _]
                  frame False {
                    n308 = Negate(x=w1094) -> (-x=w1093:i16)
                    n309 = local write "Z VEL"(w1093) -> ()
                  }
                  frame True {
                  }
                }
              }
              frame True {
                n310 = local read "Z VEL"() -> (w1095:i16)
                n311 = Greater?(x=w1095, y=i16 0) -> (0:w1096:bool)
                n312 = case shown="True" w1096 {
                  tunnel: w1095 -> [_ w1099]
                  frame False {
                  }
                  frame True {
                    n313 = Negate(x=w1099) -> (-x=w1098:i16)
                    n314 = local write "Z VEL"(w1098) -> ()
                  }
                }
              }
            }
            n315 = case shown="True" w1055 {
              frame False {
                n316 = local read "V2 VEl"() -> (w1070:i16)
                n317 = Greater?(x=w1070, y=i16 0) -> (0:w1071:bool)
                n318 = case shown="False" w1071 {
                  tunnel: w1070 -> [w1074 _]
                  frame False {
                    n319 = Negate(x=w1074) -> (-x=w1073:i16)
                    n320 = local write "V2 VEl"(w1073) -> ()
                  }
                  frame True {
                  }
                }
              }
              frame True {
                n321 = local read "V2 VEl"() -> (w1075:i16)
                n322 = Greater?(x=w1075, y=i16 0) -> (0:w1076:bool)
                n323 = case shown="True" w1076 {
                  tunnel: w1075 -> [_ w1079]
                  frame False {
                  }
                  frame True {
                    n324 = Negate(x=w1079) -> (-x=w1078:i16)
                    n325 = local write "V2 VEl"(w1078) -> ()
                  }
                }
              }
            }
          }
          frame #4 {
            n326 = local read "DIO0"() -> (w1120:bool)
            n327 = local read "StopMoveZ"() -> (w1125:bool)
            n328 = local read "StopMoveX"() -> (w1127:bool)
            n329 = local read "StopMoveV2"() -> (w1124:bool)
            n330 = local read "StopMoveY"() -> (w1126:bool)
            n331 = global read "Tick Count.vi" "Tick Count"() -> (w1129:u64)
            n332 = local read "Move Z Picomotor"() -> (w1121:bool)
            n333 = local read "Stop Hold Position"() -> (w1122:bool)
            n334 = xnode "FPGA I/O Node"("Connector1/DIO0"=w1120) -> ()  [unwired: 1 in, 1 out]
            n335 = local read "StopMoveV"() -> (w1128:bool)
            "TraceRetraceFirstUse" <- FALSE ("Boolean")
          }
        }
        n336 = case shown="True" w205 {
          frame False {
          }
          frame True {
            n337 = flat-sequence {
              frame #0 {
                n338 = local read "Move Z Picomotor Direction"() -> (w215:bool)
                n339 = Select(t=i16 4915 ("LineNumber"), s=w215, f=i16 -4915 ("LineNumber")) -> (s? t:f=w214:i16)
                n340 = xnode "FPGA I/O Node"("Connector1/AO7"=w214) -> ()  [unwired: 1 in, 1 out]
              }
              frame #1 {
                n341 = while {
                  stop <- w218 stop-if-true
                  n342 = local read "Stop Hold Position"() -> (w222:bool)
                  n343 = local read "Internal Pause"() -> (w221:bool)
                  n344 = local read "External Pause"() -> (w220:bool)
                  n345 = Or(x=w220, y=w221) -> (x .or. y?=w219:bool)
                  n346 = Or(x=w222, y=w219) -> (x .or. y?=w218:bool)
                }
              }
              frame #2 {
                n347 = xnode "FPGA I/O Node"("Connector1/AO7"=i16 0 ("LineNumber")) -> ()  [unwired: 1 in, 1 out]
              }
            }
          }
        }
        n348 = case shown="False" w207 {
          tunnel: w206 -> [w269 _]
          frame False {
            n349 = while {
              tunnel: w269 -> [w277]
              stop <- w273 stop-if-true
              n350 = local read "HoldTimer (ticks)"() -> (w279:u64)
              n351 = global read "Tick Count.vi" "Tick Count"() -> (w278:u64)
              n352 = Subtract(x=w278, y=w277) -> (x-y=w276:u64)
              n353 = Greater Than 0?(x=w279) -> (x > 0?=w280:bool)
              n354 = local read "Feedback1 on  Hold"() -> (w270:bool)
              n355 = case shown="True" w280 {
                tunnel: [FALSE w284] -> w271
                tunnel: w279 -> [_ w283]
                tunnel: w276 -> [_ w282]
                frame False {
                }
                frame True {
                  n356 = Greater?(x=w282, y=w283) -> (0:w284:bool)
                }
              }
              "HasHeldHoldTimeHappend?" <- w271
              n357 = local read "External Stop"() -> (w274:bool)
              n358 = local read "Feedback1 Boolean"() -> (w275:bool)
              n359 = Select(t=w275, s=w270, f=w271) -> (s? t:f=w272:bool)
              n360 = Compound Arithmetic op=OR(w272, w274) -> (w273:bool)
              n361 = local write "Stop Hold Position"(w273) -> ()
            }
          }
          frame True {
          }
        }
        n362 = while {
          tunnel: w206 -> [_]
          stop <- w231 stop-if-true
          n363 = local read "FeedBackType"() -> (w243:u8)
          n364 = local read "FeedBackType 2"() -> (w241:u8)
          n365 = local read "Feedback_Threshold"() -> (w228:i32)
          n366 = case shown="1" w243 {
            tunnel: [w263 w264 w265 w266 w267 w268] -> w244
            frame 0, Default {
              n367 = local read "Ext amp"() -> (w263:i16)
            }
            frame 1 {
              n368 = local read "MeasuredCurrent"() -> (w264:i16)
            }
            frame 2 {
              n369 = local read "MeasuredCurrent 2"() -> (w265:i16)
            }
            frame 3 {
              n370 = local read "Ext Phase"() -> (w266:i16)
            }
            frame 4 {
              n371 = local read "MeasuredCurrent"() -> (w267:i16)
            }
            frame 5 {
              n372 = local read "MeasuredCurrent 2"() -> (w268:i16)
            }
          }
          n373 = local read "Feedback_Threshold 2"() -> (w225:i32)
          n374 = case shown="1" w241 {
            tunnel: [w251 w252 w253 w254 w255 w256] -> w239
            frame 0, Default {
              n375 = local read "Ext amp"() -> (w251:i16)
            }
            frame 4 {
              n376 = local read "MeasuredCurrent 3"() -> (w252:i16)
            }
            frame 5 {
              n377 = local read "MeasuredCurrent 4"() -> (w253:i16)
            }
            frame 1 {
              n378 = local read "MeasuredCurrent"() -> (w254:i16)
            }
            frame 2 {
              n379 = local read "MeasuredCurrent 2"() -> (w255:i16)
            }
            frame 3 {
              n380 = local read "Ext Phase"() -> (w256:i16)
            }
          }
          n381 = To Long Integer(number=w244) -> (32bit integer=w229:i32)
          n382 = To Long Integer(number=w239) -> (32bit integer=w226:i32)
          n383 = case shown="True" "GreaterThan" {
            tunnel: w229 -> [w259 w262]
            tunnel: w228 -> [w258 w260]
            tunnel: [w257 w261] -> w238
            frame False {
              n384 = Less?(x=w259, y=w258) -> (x < y?=w257:bool)
            }
            frame True {
              n385 = Greater?(x=w262, y=w260) -> (0:w261:bool)
            }
          }
          n386 = case shown="True" "GreaterThan 2" {
            tunnel: w226 -> [w247 w250]
            tunnel: w225 -> [w246 w248]
            tunnel: [w245 w249] -> w237
            frame False {
              n387 = Less?(x=w247, y=w246) -> (x < y?=w245:bool)
            }
            frame True {
              n388 = Greater?(x=w250, y=w248) -> (0:w249:bool)
            }
          }
          n389 = Subtract(x=w226, y=w225) -> (x-y=w224:i32)
          n390 = local write "Feedback1 Boolean"(w238) -> ()
          n391 = Subtract(x=w229, y=w228) -> (x-y=w227:i32)
          n392 = local write "Feedback2 Error"(w224) -> ()
          n393 = local write "Feedback2 Boolean"(w237) -> ()
          n394 = local write "Feedback1 Error"(w227) -> ()
          n395 = local read "Stop Hold Position"() -> (w230:bool)
          n396 = local read "StopMoveV"() -> (w233:bool)
          n397 = local read "StopMoveZ"() -> (w234:bool)
          n398 = local read "StopMoveX"() -> (w236:bool)
          n399 = local read "StopMoveY"() -> (w235:bool)
          n400 = local read "StopMoveV2"() -> (w232:bool)
          n401 = Compound Arithmetic op=AND(w230, w236, w235, w234, w233, w232) -> (w231:bool)
        }
        n402 = case shown="False" w212 {
          tunnel: w206 -> [w853 _]
          frame False {
            n403 = while {
              shift-right: [w855] -> _
              shift-left: w853 -> [w858]
              stop <- w854 stop-if-true
              n404 = flat-sequence {
                tunnel: w858 -> [w860]
                tunnel: [w861] -> w859
                tunnel: w859 -> [w886]
                tunnel: [w886] -> w857
                tunnel: [w882] -> w856
                tunnel: [w917] -> w855
                tunnel: w857 -> [w917]
                tunnel: w856 -> [w911]
                tunnel: [w912] -> w854
                frame #0 {
                  n405 = local read "Internal Pause"() -> (w863:bool)
                  n406 = local read "External Pause"() -> (w864:bool)
                  n407 = Or(x=w864, y=w863) -> (x .or. y?=w862:bool)
                  n408 = case shown="True" w862 {
                    tunnel: w860 -> [w865 w868]
                    tunnel: [w865 w866] -> w861
                    frame False {
                    }
                    frame True {
                      n409 = global read "Tick Count.vi" "Tick Count"() -> (w867:u64)
                      n410 = while {
                        shift-right: [w880] -> w866
                        shift-left: w868 -> [w872]
                        shift-right: [w875] -> _
                        shift-left: w867 -> [w874]
                        stop <- w869 stop-if-true
                        n411 = local read "External Pause"() -> (w879:bool)
                        n412 = local read "Internal Pause"() -> (w877:bool)
                        n413 = global read "Tick Count.vi" "Tick Count"() -> (w875:u64)
                        n414 = local read "External Stop"() -> (w871:bool)
                        n415 = Not(x=w879) -> (.not. x?=w878:bool)
                        n416 = Not(x=w877) -> (.not. x?=w876:bool)
                        n417 = Subtract(x=w875, y=w874) -> (x-y=w873:u64)
                        n418 = And(x=w878, y=w876) -> (x .and. y?=w870:bool)
                        n419 = Add(x=w873, y=w872) -> (x+y=w880:u64)
                        n420 = Or(x=w870, y=w871) -> (x .or. y?=w869:bool)
                      }
                    }
                  }
                }
                frame #1 {
                  n421 = global read "Tick Count.vi" "Tick Count"() -> (w885:u64)
                  n422 = Subtract(x=w885, y=w886) -> (x-y=w883:u64)
                  n423 = To Fixed-Point(number=w883) -> (fixed-point=w884:fxp<+,64,64>)  [unwired: 1 in]
                  n424 = case shown="True" "Change V on Fly" {
                    tunnel: w884 -> [w894 _]
                    tunnel: [w893 FALSE ("Finished Move")] -> w882
                    frame False {
                      n425 = local read "Jump V"() -> (w892:bool)
                      n426 = local read "V END"() -> (w891:i16)
                      n427 = case shown="True" w892 {
                        tunnel: w891 -> [w903 w904]
                        tunnel: [w902 w904] -> w889
                        tunnel: w894 -> [w901 _]
                        tunnel: [w900 TRUE ("Finished Move")] -> w893
                        frame False {
                          n428 = local read "ExpandVelScaller V"() -> (w895:i16)
                          n429 = local read "V VEl"() -> (w898:i16)
                          n430 = local read "V START"() -> (w899:i16)
                          n431 = Number To Boolean Array(number=w898) -> (Boolean array=w897:bool[])
                          n432 = Boolean Array To Number(Boolean array=w897) -> (number=w896:fxp<+/-,16,16>)
                          n433 = call "LinearMove.vi"("Time"=w901, "Start"=w899, "End"=w903, "Velocity"=w896, "ExpandVelScaller"=w895) -> ("OutPosition"=w902:i16, "Finished Move"=w900:bool)  [unwired: 13 in]
                        }
                        frame True {
                        }
                      }
                      n434 = local read "Invert AO3 Output (V1)"() -> (w887:bool)
                      n435 = Negate(x=w889) -> (-x=w888:i16)
                      n436 = local write "Applied Voltage"(w889) -> ()
                      n437 = Select(t=w888, s=w887, f=w889) -> (s? t:f=w890:i16)
                      n438 = xnode "FPGA I/O Node"("Connector1/AO3"=w890) -> ()  [unwired: 1 in, 1 out]
                    }
                    frame True {
                      n439 = local read "Invert AO3 Output (V1)"() -> (w908:bool)
                      n440 = local write "Applied Voltage"("V on Fly") -> ()
                      n441 = Negate(x="V on Fly") -> (-x=w909:i16)
                      n442 = Select(t=w909, s=w908, f="V on Fly") -> (s? t:f=w906:i16)
                      n443 = xnode "FPGA I/O Node"("Connector1/AO3"=w906) -> ()  [unwired: 1 in, 1 out]
                    }
                  }
                }
                frame #2 {
                  n444 = local read "OnlyStopLineONCE V"() -> (w913:bool)
                  n445 = case shown="False" w913 {
                    tunnel: [w918 FALSE ("EndCurrentLine")] -> w914
                    frame False {
                      n446 = local read "EndCurrentLine"() -> (w918:bool)
                      n447 = case shown="True" w918 {
                        frame False {
                        }
                        frame True {
                          n448 = local write "OnlyStopLineONCE V"(TRUE ("EndCurrentLine")) -> ()
                        }
                      }
                    }
                    frame True {
                    }
                  }
                  n449 = local read "External Stop"() -> (w915:bool)
                  n450 = Or(x=w911, y=w914) -> (x .or. y?=w916:bool)
                  n451 = Or(x=w915, y=w916) -> (x .or. y?=w912:bool)
                }
              }
              n452 = local write "StopMoveV"(w854) -> ()
            }
          }
          frame True {
          }
        }
        n453 = case shown="False" w211 {
          tunnel: w206 -> [w800 _]
          frame False {
            n454 = while {
              shift-right: [w802] -> _
              shift-left: w800 -> [w805]
              stop <- w801 stop-if-true
              n455 = flat-sequence {
                tunnel: w805 -> [w807]
                tunnel: [w808] -> w806
                tunnel: w806 -> [w842]
                tunnel: [w842] -> w804
                tunnel: [w839] -> w803
                tunnel: [w849] -> w802
                tunnel: w804 -> [w849]
                tunnel: w803 -> [w843]
                tunnel: [w844] -> w801
                frame #0 {
                  n456 = local read "Internal Pause"() -> (w810:bool)
                  n457 = local read "External Pause"() -> (w811:bool)
                  n458 = Or(x=w811, y=w810) -> (x .or. y?=w809:bool)
                  n459 = case shown="True" w809 {
                    tunnel: w807 -> [w812 w815]
                    tunnel: [w812 w813] -> w808
                    frame False {
                    }
                    frame True {
                      n460 = global read "Tick Count.vi" "Tick Count"() -> (w814:u64)
                      n461 = while {
                        shift-right: [w827] -> w813
                        shift-left: w815 -> [w819]
                        shift-right: [w822] -> _
                        shift-left: w814 -> [w821]
                        stop <- w816 stop-if-true
                        n462 = local read "External Pause"() -> (w826:bool)
                        n463 = local read "Internal Pause"() -> (w824:bool)
                        n464 = global read "Tick Count.vi" "Tick Count"() -> (w822:u64)
                        n465 = local read "External Stop"() -> (w818:bool)
                        n466 = Not(x=w826) -> (.not. x?=w825:bool)
                        n467 = Not(x=w824) -> (.not. x?=w823:bool)
                        n468 = Subtract(x=w822, y=w821) -> (x-y=w820:u64)
                        n469 = And(x=w825, y=w823) -> (x .and. y?=w817:bool)
                        n470 = Add(x=w820, y=w819) -> (x+y=w827:u64)
                        n471 = Or(x=w817, y=w818) -> (x .or. y?=w816:bool)
                      }
                    }
                  }
                }
                frame #1 {
                  # "MAE 18/8/2014: Changed 0 to -32768 to allow -10 to 10V option. Note: as this is the full range of an I16 the coercion isn't doing much. In future make this boolean controlled from the T/F in advanced settings"
                  n472 = global read "Tick Count.vi" "Tick Count"() -> (w841:u64)
                  n473 = Subtract(x=w841, y=w842) -> (x-y=w828:u64)
                  n474 = To Fixed-Point(number=w828) -> (fixed-point=w840:fxp<+,64,64>)  [unwired: 1 in]
                  n475 = local read "X VEL"() -> (w832:i16)
                  n476 = local read "ExpandVelScaller X"() -> (w829:i16)
                  n477 = local read "X END"() -> (w830:i16)
                  n478 = local read "X START"() -> (w831:i16)
                  n479 = Number To Boolean Array(number=w832) -> (Boolean array=w838:bool[])
                  n480 = Boolean Array To Number(Boolean array=w838) -> (number=w837:fxp<+/-,16,16>)
                  n481 = call "LinearMove.vi"("Time"=w840, "Start"=w831, "End"=w830, "Velocity"=w837, "ExpandVelScaller"=w829) -> ("OutPosition"=w833:i16, "Finished Move"=w839:bool)  [unwired: 13 in]
                  n482 = In Range and Coerce(upper limit=i16 32767, x=w833, lower limit=i16 -32768) -> (coerced(x)=w834:i16)  [unwired: 1 out]
                  n483 = local write "Applied X"(w834) -> ()
                  n484 = xnode "FPGA I/O Node"("Connector1/AO0"=w834) -> ()  [unwired: 1 in, 1 out]
                }
                frame #2 {
                  n485 = local read "OnlyStopLineONCE X"() -> (w846:bool)
                  n486 = case shown="False" w846 {
                    tunnel: [w850 FALSE ("EndCurrentLine")] -> w845
                    frame False {
                      n487 = local read "EndCurrentLine"() -> (w850:bool)
                      n488 = case shown="True" w850 {
                        frame False {
                        }
                        frame True {
                          n489 = local write "OnlyStopLineONCE X"(TRUE ("EndCurrentLine")) -> ()
                        }
                      }
                    }
                    frame True {
                    }
                  }
                  n490 = local read "External Stop"() -> (w848:bool)
                  n491 = Or(x=w843, y=w845) -> (x .or. y?=w847:bool)
                  n492 = Or(x=w848, y=w847) -> (x .or. y?=w844:bool)
                }
              }
              n493 = local write "StopMoveX"(w801) -> ()
            }
          }
          frame True {
          }
        }
        n494 = case shown="False" w210 {
          tunnel: w206 -> [w747 _]
          frame False {
            n495 = while {
              shift-right: [w749] -> _
              shift-left: w747 -> [w752]
              stop <- w748 stop-if-true
              n496 = flat-sequence {
                tunnel: w752 -> [w754]
                tunnel: [w755] -> w753
                tunnel: w753 -> [w789]
                tunnel: [w789] -> w751
                tunnel: [w786] -> w750
                tunnel: [w796] -> w749
                tunnel: w751 -> [w796]
                tunnel: w750 -> [w790]
                tunnel: [w791] -> w748
                frame #0 {
                  n497 = local read "External Pause"() -> (w758:bool)
                  n498 = local read "Internal Pause"() -> (w757:bool)
                  n499 = Or(x=w758, y=w757) -> (x .or. y?=w756:bool)
                  n500 = case shown="True" w756 {
                    tunnel: w754 -> [w759 w762]
                    tunnel: [w759 w760] -> w755
                    frame False {
                    }
                    frame True {
                      n501 = global read "Tick Count.vi" "Tick Count"() -> (w761:u64)
                      n502 = while {
                        shift-right: [w774] -> w760
                        shift-left: w762 -> [w766]
                        shift-right: [w769] -> _
                        shift-left: w761 -> [w768]
                        stop <- w763 stop-if-true
                        n503 = local read "External Pause"() -> (w773:bool)
                        n504 = local read "Internal Pause"() -> (w771:bool)
                        n505 = global read "Tick Count.vi" "Tick Count"() -> (w769:u64)
                        n506 = local read "External Stop"() -> (w765:bool)
                        n507 = Not(x=w773) -> (.not. x?=w772:bool)
                        n508 = Not(x=w771) -> (.not. x?=w770:bool)
                        n509 = Subtract(x=w769, y=w768) -> (x-y=w767:u64)
                        n510 = And(x=w772, y=w770) -> (x .and. y?=w764:bool)
                        n511 = Add(x=w767, y=w766) -> (x+y=w774:u64)
                        n512 = Or(x=w764, y=w765) -> (x .or. y?=w763:bool)
                      }
                    }
                  }
                }
                frame #1 {
                  # "MAE 18/8/2014: Changed 0 to -32768 to allow -10 to 10V option. Note: as this is the full range of an I16 the coercion isn't doing much. In future make this boolean controlled from the T/F in advanced settings"
                  n513 = global read "Tick Count.vi" "Tick Count"() -> (w788:u64)
                  n514 = Subtract(x=w788, y=w789) -> (x-y=w775:u64)
                  n515 = To Fixed-Point(number=w775) -> (fixed-point=w787:fxp<+,64,64>)  [unwired: 1 in]
                  n516 = local read "Y VEL"() -> (w779:i16)
                  n517 = local read "ExpandVelScaller Y"() -> (w776:i16)
                  n518 = local read "Y END"() -> (w777:i16)
                  n519 = local read "Y START"() -> (w778:i16)
                  n520 = Number To Boolean Array(number=w779) -> (Boolean array=w785:bool[])
                  n521 = Boolean Array To Number(Boolean array=w785) -> (number=w784:fxp<+/-,16,16>)
                  n522 = call "LinearMove.vi"("Time"=w787, "Start"=w778, "End"=w777, "Velocity"=w784, "ExpandVelScaller"=w776) -> ("OutPosition"=w780:i16, "Finished Move"=w786:bool)  [unwired: 13 in]
                  n523 = In Range and Coerce(upper limit=i16 32767, x=w780, lower limit=i16 -32768) -> (coerced(x)=w781:i16)  [unwired: 1 out]
                  n524 = local write "Applied Y"(w781) -> ()
                  n525 = xnode "FPGA I/O Node"("Connector1/AO1"=w781) -> ()  [unwired: 1 in, 1 out]
                }
                frame #2 {
                  n526 = local read "OnlyStopLineONCE Y"() -> (w792:bool)
                  n527 = case shown="False" w792 {
                    tunnel: [w797 FALSE ("EndCurrentLine")] -> w793
                    frame False {
                      n528 = local read "EndCurrentLine"() -> (w797:bool)
                      n529 = case shown="True" w797 {
                        frame False {
                        }
                        frame True {
                          n530 = local write "OnlyStopLineONCE Y"(TRUE ("EndCurrentLine")) -> ()
                        }
                      }
                    }
                    frame True {
                    }
                  }
                  n531 = local read "External Stop"() -> (w795:bool)
                  n532 = Or(x=w790, y=w793) -> (x .or. y?=w794:bool)
                  n533 = Or(x=w795, y=w794) -> (x .or. y?=w791:bool)
                }
              }
              n534 = local write "StopMoveY"(w748) -> ()
            }
          }
          frame True {
          }
        }
        n535 = case shown="False" w209 {
          tunnel: w206 -> [w354 _]
          frame False {
            n536 = local read "Applied X"() -> (w353:i16)
            n537 = while {
              shift-right: [w358] -> _
              shift-left: w354 -> [w361]
              shift-right: [w355] -> _
              shift-left: w353 -> [w356]
              stop <- w357 stop-if-true
              n538 = flat-sequence {
                tunnel: w361 -> [w364]
                tunnel: [w365] -> w362
                tunnel: w362 -> [w402]
                tunnel: [w402] -> w360
                tunnel: [w397] -> w359
                tunnel: w356 -> [w391]
                tunnel: [w390] -> w355
                tunnel: [w743] -> w358
                tunnel: w360 -> [w743]
                tunnel: w359 -> [w737]
                tunnel: [w738] -> w357
                frame #0 {
                  n539 = local read "Update Position Loop Wait Time (ms)"() -> (w363:u16)
                  n540 = local read "External Pause"() -> (w368:bool)
                  n541 = local read "Internal Pause"() -> (w367:bool)
                  n542 = Or(x=w368, y=w367) -> (x .or. y?=w366:bool)
                  n543 = case shown="True" w366 {
                    tunnel: w364 -> [w369 w372]
                    tunnel: [w369 w370] -> w365
                    frame False {
                    }
                    frame True {
                      n544 = global read "Tick Count.vi" "Tick Count"() -> (w371:u64)
                      n545 = while {
                        shift-right: [w384] -> w370
                        shift-left: w372 -> [w376]
                        shift-right: [w379] -> _
                        shift-left: w371 -> [w378]
                        stop <- w373 stop-if-true
                        n546 = local read "External Pause"() -> (w383:bool)
                        n547 = local read "Internal Pause"() -> (w381:bool)
                        n548 = global read "Tick Count.vi" "Tick Count"() -> (w379:u64)
                        n549 = local read "External Stop"() -> (w375:bool)
                        n550 = Not(x=w383) -> (.not. x?=w382:bool)
                        n551 = Not(x=w381) -> (.not. x?=w380:bool)
                        n552 = Subtract(x=w379, y=w378) -> (x-y=w377:u64)
                        n553 = And(x=w382, y=w380) -> (x .and. y?=w374:bool)
                        n554 = Add(x=w377, y=w376) -> (x+y=w384:u64)
                        n555 = Or(x=w374, y=w375) -> (x .or. y?=w373:bool)
                      }
                    }
                  }
                  n556 = call "Loop Timer"("Count(mSec)"=w363) -> ()  [unwired: 1 out]
                }
                frame #1 {
                  # "MAE 18/8/2014: Changed 0 to -32768 to allow -10 to 10V option. Note: as this is the full range of an I16 the coercion isn't doing much. In future make this boolean controlled from the T/F in advanced settings"
                  n557 = global read "Tick Count.vi" "Tick Count"() -> (w401:u64)
                  n558 = local read "Feedback2 Boolean"() -> (w385:bool)
                  n559 = local read "LineType"() -> (w388:i16)
                  n560 = local read "Feedback1 Boolean"() -> (w386:bool)
                  n561 = Subtract(x=w401, y=w402) -> (x-y=w393:u64)
                  n562 = To Fixed-Point(number=w393) -> (fixed-point=w389:fxp<+,64,64>)  [unwired: 1 in]
                  n563 = Or(x=w386, y=w385) -> (x .or. y?=w387:bool)
                  n564 = case shown="11" w388 {
                    tunnel: "P" -> [_ _ _ w438 w450 w466 w487 _ w522 _ _ _]
                    tunnel: [w405 w415 w422 w433 w446 w461 w477 w510 w517 w539 w603 w675] -> w397
                    tunnel: [w404 w414 w424 w436 w448 w464 w476 w513 w520 w541 w605 w677] -> w396
                    tunnel: "Upper limit Of dZ" -> [_ _ _ w432 w447 w463 w486 _ w516 _ _ _]
                    tunnel: w391 -> [_ _ _ _ _ _ w484 _ _ _ _ _]
                    tunnel: [_ _ _ _ _ _ w483 _ _ _ _ _] -> w390
                    tunnel: w389 -> [w403 w413 w423 _ _ _ _ _ _ w540 w604 w676]
                    tunnel: w387 -> [_ w412 w422 _ _ _ _ _ _ _ _ _]
                    tunnel: w385 -> [_ _ _ _ _ _ _ _ w515 _ _ _]
                    frame 0, Default {
                      # "Normal Move"
                      n565 = local read "Z VEL"() -> (w408:i16)
                      n566 = local read "ExpandVelScaller Z"() -> (w411:i16)
                      n567 = local read "Z END"() -> (w410:i16)
                      n568 = local read "Z START"() -> (w409:i16)
                      n569 = Number To Boolean Array(number=w408) -> (Boolean array=w406:bool[])
                      n570 = Boolean Array To Number(Boolean array=w406) -> (number=w407:fxp<+/-,16,16>)
                      n571 = call "LinearMove.vi"("Time"=w403, "Start"=w409, "End"=w410, "Velocity"=w407, "ExpandVelScaller"=w411) -> ("OutPosition"=w404:i16, "Finished Move"=w405:bool)  [unwired: 13 in]
                    }
                    frame 1 {
                      # "Pause on Set Point"
                      n572 = local write "Internal Pause"(w412) -> ()
                      n573 = local read "Z VEL"() -> (w418:i16)
                      n574 = local read "ExpandVelScaller Z"() -> (w421:i16)
                      n575 = local read "Z END"() -> (w420:i16)
                      n576 = local read "Z START"() -> (w419:i16)
                      n577 = Number To Boolean Array(number=w418) -> (Boolean array=w416:bool[])
                      n578 = Boolean Array To Number(Boolean array=w416) -> (number=w417:fxp<+/-,16,16>)
                      n579 = call "LinearMove.vi"("Time"=w413, "Start"=w419, "End"=w420, "Velocity"=w417, "ExpandVelScaller"=w421) -> ("OutPosition"=w414:i16, "Finished Move"=w415:bool)  [unwired: 13 in]
                    }
                    frame 2 {
                      # "STOP Current Move on SetPoint"
                      n580 = local read "Z VEL"() -> (w427:i16)
                      n581 = local read "ExpandVelScaller Z"() -> (w430:i16)
                      n582 = local read "Z END"() -> (w429:i16)
                      n583 = local read "Z START"() -> (w428:i16)
                      n584 = Number To Boolean Array(number=w427) -> (Boolean array=w425:bool[])
                      n585 = Boolean Array To Number(Boolean array=w425) -> (number=w426:fxp<+/-,16,16>)
                      n586 = call "LinearMove.vi"("Time"=w423, "Start"=w428, "End"=w429, "Velocity"=w426, "ExpandVelScaller"=w430) -> ("OutPosition"=w424:i16)  [unwired: 13 in, 1 out]
                    }
                    frame 4 {
                      # "For scanning-Propotional Controller for constant distance scanning"
                      n587 = local read "Feedback1 Error"() -> (w431:i32)
                      n588 = Multiply(x=w438, y=w431) -> (x*y=w443:fxp<+/-,64,33>)
                      n589 = To Word Integer(number=w443) -> (16bit integer=w442:i16)
                      n590 = To Long Integer(number=w442) -> (32bit integer=w444:i32)
                      n591 = local read "StopMoveY"() -> (w434:bool)
                      n592 = local read "StopMoveX"() -> (w435:bool)
                      n593 = local read "Applied Z"() -> (w437:i16)
                      n594 = Negate(x=w432) -> (-x=w439:i32)
                      n595 = And(x=w435, y=w434) -> (x .and. y?=w433:bool)
                      n596 = In Range and Coerce(upper limit=w432, x=w444, lower limit=w439) -> (coerced(x)=w440:i32)  [unwired: 1 out]
                      n597 = To Long Integer(number=w437) -> (32bit integer=w441:i32)
                      n598 = Add(x=w441, y=w440) -> (x+y=w436:i32)
                    }
                    frame 11 {
                      # "Dependent on hold time-Propotional Controller for constant distance scanning"
                      n599 = local read "Feedback1 Error"() -> (w445:i32)
                      n600 = Multiply(x=w450, y=w445) -> (x*y=w455:fxp<+/-,64,33>)
                      n601 = To Word Integer(number=w455) -> (16bit integer=w454:i16)
                      n602 = To Long Integer(number=w454) -> (32bit integer=w456:i32)
                      n603 = local read "HasHeldHoldTimeHappend?"() -> (w446:bool)
                      n604 = local read "Applied Z"() -> (w449:i16)
                      n605 = Negate(x=w447) -> (-x=w451:i32)
                      n606 = In Range and Coerce(upper limit=w447, x=w456, lower limit=w451) -> (coerced(x)=w452:i32)  [unwired: 1 out]
                      n607 = To Long Integer(number=w449) -> (32bit integer=w453:i32)
                      n608 = Add(x=w453, y=w452) -> (x+y=w448:i32)
                    }
                    frame 10 {
                      # "deciding the limit of the Z movement (up or down) regardless of the x value"
                      # "convert the difference in siganls to distance in um"
                      # "External signal-Feedback_Threshold"
                      # "Dependent on holdtime-Propotional Controller for constant distance scanning ONLY for POSITIVE"
                      n609 = local read "Feedback1 Error"() -> (w457:i32)
                      n610 = Multiply(x=w466, y=w457) -> (x*y=w470:fxp<+/-,64,33>)
                      n611 = To Word Integer(number=w470) -> (16bit integer=w469:i16)
                      n612 = To Long Integer(number=w469) -> (32bit integer=w471:i32)
                      n613 = Negate(x=w463) -> (-x=w467:i32)
                      n614 = In Range and Coerce(upper limit=w463, x=w471, lower limit=w467) -> (coerced(x)=w459:i32)  [unwired: 1 out]
                      n615 = Less?(x=w459, y=0) -> (x < y?=w460:bool)
                      n616 = local read "HasHeldHoldTimeHappend?"() -> (w461:bool)
                      n617 = case shown="True" w460 {
                        tunnel: w459 -> [_ w473]
                        tunnel: [0 w473] -> w462
                        frame False {
                        }
                        frame True {
                        }
                      }
                      n618 = local read "Applied Z"() -> (w465:i16)
                      n619 = To Long Integer(number=w465) -> (32bit integer=w468:i32)
                      n620 = Add(x=w468, y=w462) -> (x+y=w464:i32)
                    }
                    frame 5 {
                      # "Proportional controller for constant distance scanning - with storing the positions in a buffer"
                      n621 = local read "Feedback1 Error"() -> (w474:i32)
                      n622 = local read "TraceRetraceFirstUse"() -> (w475:bool)
                      n623 = local read "Applied X"() -> (w483:i16)
                      n624 = local read "Applied Z"() -> (w485:i16)
                      n625 = Multiply(x=w487, y=w474) -> (x*y=w489:fxp<+/-,64,33>)
                      n626 = To Word Integer(number=w489) -> (16bit integer=w490:i16)
                      n627 = Subtract(x=w483, y=w484) -> (x-y=w482:i16)
                      n628 = To Long Integer(number=w490) -> (32bit integer=w488:i32)
                      n629 = case shown="False" w475 {
                        tunnel: w482 -> [w502 w505]
                        tunnel: [w501 w505] -> w481
                        tunnel: [w500 w504] -> w480
                        tunnel: w484 -> [w500 w503]
                        frame False {
                          n630 = Increment(x=w502) -> (x+1=w501:i16)
                        }
                        frame True {
                          n631 = Increment(x=w503) -> (x+1=w504:i16)
                        }
                      }
                      n632 = Negate(x=w486) -> (-x=w493:i32)
                      n633 = In Range and Coerce(upper limit=w486, x=w488, lower limit=w493) -> (coerced(x)=w492:i32)  [unwired: 1 out]
                      n634 = To Long Integer(number=w485) -> (32bit integer=w491:i32)
                      n635 = Add(x=w491, y=w492) -> (x+y=w476:i32)
                      n636 = for {
                        N: w481 -> [_]
                        shift-right: [w495] -> _
                        shift-left: w480 -> [w496]
                        tunnel: w476 -> [w499]
                        n637 = To Unsigned Long Integer(number=w496) -> (unsigned 32bit integer=w497:u32)
                        n638 = To Word Integer(number=w499) -> (16bit integer=w498:i16)
                        n639 = local write "TraceRetraceFirstUse"(TRUE ("TraceRetraceFirst?")) -> ()
                        n640 = xnode ("Memory Write")("Address"=w497, "Data"=w498) -> ()  [unwired: 1 in, 1 out]
                        n641 = Increment(x=w496) -> (x+1=w495:i16)
                      }
                      n642 = local read "StopMoveY"() -> (w478:bool)
                      n643 = local read "StopMoveX"() -> (w479:bool)
                      n644 = And(x=w479, y=w478) -> (x .and. y?=w477:bool)
                    }
                    frame 6 {
                      # "retrace the Z positions stored in the buffer, see feedbaack type 5"
                      n645 = local read "Applied X"() -> (w506:i16)
                      n646 = To Unsigned Long Integer(number=w506) -> (unsigned 32bit integer=w509:u32)
                      n647 = Add(x="Xoffset", y=w509) -> (x+y=w507:u32)
                      n648 = xnode ("Memory Read")("Address"=w507) -> ("Data"=w513:i16)  [unwired: 1 in, 1 out]
                      n649 = local read "StopMoveY"() -> (w511:bool)
                      n650 = local read "StopMoveX"() -> (w512:bool)
                      n651 = And(x=w512, y=w511) -> (x .and. y?=w510:bool)
                    }
                    frame 7 {
                      # "Proportianal controller for constant distance scan, with ability to pause based on a secondary signal"
                      n652 = local write "Internal Pause"(w515) -> ()
                      n653 = local read "Feedback1 Error"() -> (w514:i32)
                      n654 = Multiply(x=w522, y=w514) -> (x*y=w527:fxp<+/-,64,33>)
                      n655 = To Word Integer(number=w527) -> (16bit integer=w526:i16)
                      n656 = To Long Integer(number=w526) -> (32bit integer=w528:i32)
                      n657 = local read "StopMoveY"() -> (w518:bool)
                      n658 = local read "StopMoveX"() -> (w519:bool)
                      n659 = local read "Applied Z"() -> (w521:i16)
                      n660 = Negate(x=w516) -> (-x=w523:i32)
                      n661 = And(x=w519, y=w518) -> (x .and. y?=w517:bool)
                      n662 = In Range and Coerce(upper limit=w516, x=w528, lower limit=w523) -> (coerced(x)=w524:i32)  [unwired: 1 out]
                      n663 = To Long Integer(number=w521) -> (32bit integer=w525:i32)
                      n664 = Add(x=w525, y=w524) -> (x+y=w520:i32)
                    }
                    frame 8 {
                      # "Sum of most recent 1024"
                      n665 = local read "FeedBackType"() -> (w531:u8)
                      n666 = local read "Count Average"() -> (w532:i16)
                      n667 = case shown="1" w531 {
                        tunnel: [w544 w545 w546 w547 w548 w549] -> w530
                        frame 0, Default {
                          n668 = local read "Ext amp"() -> (w544:i16)
                        }
                        frame 1 {
                          n669 = local read "MeasuredCurrent"() -> (w545:i16)
                        }
                        frame 2 {
                          n670 = local read "MeasuredCurrent 2"() -> (w546:i16)
                        }
                        frame 3 {
                          n671 = local read "Ext Phase"() -> (w547:i16)
                        }
                        frame 4 {
                          n672 = local read "MeasuredCurrent"() -> (w548:i16)
                        }
                        frame 5 {
                          n673 = local read "MeasuredCurrent 2"() -> (w549:i16)
                        }
                      }
                      n674 = Equal?(x=w532, y="P2AvgWhole") -> (x = y?=w542:bool)
                      n675 = local read "ExtraTime 2"() -> (w535:fxp<+,64,64>)
                      n676 = To Long Integer(number=w530) -> (32bit integer=w529:i32)
                      n677 = local read "AverageSum"() -> (w538:i64)
                      n678 = case shown="True" w542 {
                        tunnel: w529 -> [w558 w578]
                        tunnel: w538 -> [w559 w585]
                        tunnel: [w560 w585] -> w543
                        tunnel: w532 -> [w557 w572]
                        tunnel: [w556 w572] -> w537
                        tunnel: [w555 w586] -> w541
                        tunnel: w540 -> [w553 w580]
                        tunnel: [FALSE w574] -> w539
                        tunnel: [w553 w582] -> w536
                        tunnel: w535 -> [_ w582]
                        tunnel: [w550 w570] -> w534
                        frame False {
                          n679 = local read "SampleIterator"() -> (w550:i16)
                          n680 = local read "IterateHolder"() -> (w552:i16)
                          n681 = Less?(x=w550, y=w552) -> (x < y?=w551:bool)
                          n682 = case shown="True" w551 {
                            tunnel: [w561 w568] -> w560
                            tunnel: w559 -> [w561 w567]
                            tunnel: w558 -> [_ w563]
                            tunnel: w557 -> [w562 w565]
                            tunnel: [w562 w566] -> w556
                            frame False {
                            }
                            frame True {
                              # "Count up to 1024 (start at 0) data points then start moving"
                              n683 = To Quad Integer(1:w563) -> (0:w564:i64)
                              n684 = Increment(x=w565) -> (x+1=w566:i16)
                              n685 = Add(x=w567, y=w564) -> (x+y=w568:i64)
                            }
                          }
                          n686 = local read "Applied Z"() -> (w555:i16)
                        }
                        frame True {
                          # "STOP Current Move on SetPoint"
                          n687 = local read "AverageSum"() -> (w584:i64)
                          n688 = local read "Feedback_Threshold"() -> (w569:i32)
                          n689 = Subtract(x=w580, y=w582) -> (x-y=w583:fxp<+/-,64,65>)
                          n690 = Scale By Power Of 2(n="P2AvgMinus", x=w584) -> (x*2^n=w573:i64)
                          n691 = To Fixed-Point(fixed-point type=w580, number=w583) -> (fixed-point=w581:fxp<+,64,64>)
                          n692 = local read "Z VEL"() -> (w589:i16)
                          n693 = Subtract(x=w573, y=w569) -> (x-y=w579:i64)
                          n694 = local read "ExpandVelScaller Z"() -> (w592:i16)
                          n695 = local read "Z END"() -> (w591:i16)
                          n696 = local read "Z START"() -> (w590:i16)
                          n697 = Number To Boolean Array(number=w589) -> (Boolean array=w587:bool[])
                          n698 = Add(x=w569, y=w573) -> (x+y=w577:i64)
                          n699 = Boolean Array To Number(Boolean array=w587) -> (number=w588:fxp<+/-,16,16>)
                          n700 = Greater?(x=w578, y=w577) -> (0:w576:bool)
                          n701 = call "LinearMove.vi"("Time"=w581, "Start"=w590, "End"=w591, "Velocity"=w588, "ExpandVelScaller"=w592) -> ("OutPosition"=w586:i16)  [unwired: 13 in, 1 out]
                          n702 = Less?(x=w578, y=w579) -> (x < y?=w575:bool)
                          n703 = Or(x=w576, y=w575) -> (x .or. y?=w574:bool)
                          n704 = local read "SampleNum"() -> (w570:i16)
                        }
                      }
                      "ExtraTime 2" <- w536
                      n705 = local write "IterateHolder"(w534) -> ()
                      n706 = local write "AverageSum"(w543) -> ()
                      n707 = local write "Count Average"(w537) -> ()
                    }
                    frame 9 {
                      # "Sum of most recent 1024"
                      n708 = local read "FeedBackType"() -> (w595:u8)
                      n709 = local read "P2AvgWhole"() -> (w596:i32)
                      n710 = local read "Count Average"() -> (w600:i16)
                      n711 = case shown="1" w595 {
                        tunnel: [w608 w609 w610 w611 w612 w613] -> w594
                        frame 0, Default {
                          n712 = local read "Ext amp"() -> (w608:i16)
                        }
                        frame 1 {
                          n713 = local read "MeasuredCurrent"() -> (w609:i16)
                        }
                        frame 2 {
                          n714 = local read "MeasuredCurrent 2"() -> (w610:i16)
                        }
                        frame 3 {
                          n715 = local read "Ext Phase"() -> (w611:i16)
                        }
                        frame 4 {
                          n716 = local read "MeasuredCurrent"() -> (w612:i16)
                        }
                        frame 5 {
                          n717 = local read "MeasuredCurrent 2"() -> (w613:i16)
                        }
                      }
                      n718 = Equal?(x=w600, y=w596) -> (x = y?=w606:bool)
                      n719 = local read "ExtraTime 3"() -> (w598:fxp<+,64,64>)
                      n720 = To Long Integer(number=w594) -> (32bit integer=w593:i32)
                      n721 = local read "AverageSum"() -> (w602:i64)
                      n722 = case shown="True" w606 {
                        tunnel: w593 -> [w622 w634]
                        tunnel: w602 -> [w623 _]
                        tunnel: [w624 w636] -> w607
                        tunnel: w600 -> [w621 w642]
                        tunnel: [w620 w642] -> w601
                        tunnel: [w619 w652] -> w605
                        tunnel: w604 -> [w617 w648]
                        tunnel: [FALSE w643] -> w603
                        tunnel: [w617 w650] -> w599
                        tunnel: w598 -> [_ w650]
                        tunnel: [w614 w639] -> w597
                        frame False {
                          n723 = local read "SampleIterator"() -> (w614:i16)
                          n724 = local read "IterateHolder"() -> (w616:i16)
                          n725 = Less?(x=w614, y=w616) -> (x < y?=w615:bool)
                          n726 = case shown="True" w615 {
                            tunnel: [w625 w632] -> w624
                            tunnel: w623 -> [w625 w631]
                            tunnel: w622 -> [_ w630]
                            tunnel: w621 -> [w626 w628]
                            tunnel: [w626 w627] -> w620
                            frame False {
                            }
                            frame True {
                              # "Count up to 1024 (start at 0) data points then start moving"
                              n727 = To Quad Integer(1:w630) -> (0:w629:i64)
                              n728 = Increment(x=w628) -> (x+1=w627:i16)
                              n729 = Add(x=w631, y=w629) -> (x+y=w632:i64)
                            }
                          }
                          n730 = local read "Applied Z"() -> (w619:i16)
                        }
                        frame True {
                          # "STOP Current Move on SetPoint"
                          n731 = local read "AverageSum"() -> (w638:i64)
                          n732 = local read "P2AvgMinus"() -> (w635:i32)
                          n733 = local read "Feedback_Threshold"() -> (w633:i32)
                          n734 = Subtract(x=w648, y=w650) -> (x-y=w651:fxp<+/-,64,65>)
                          n735 = Scale By Power Of 2(n=w635, x=w638) -> (x*2^n=w637:i64)
                          n736 = Subtract(x=w637, y=w633) -> (x-y=w647:i64)
                          n737 = local read "SampleIterator"() -> (w639:i16)
                          n738 = To Fixed-Point(fixed-point type=w648, number=w651) -> (fixed-point=w649:fxp<+,64,64>)
                          n739 = local read "IterateHolder"() -> (w641:i16)
                          n740 = Add(x=w633, y=w637) -> (x+y=w646:i64)
                          n741 = local read "Z VEL"() -> (w655:i16)
                          n742 = Less?(x=w639, y=w641) -> (x < y?=w640:bool)
                          "x < y?" <- w640
                          n743 = Greater?(x=w634, y=w646) -> (0:w645:bool)
                          n744 = local read "ExpandVelScaller Z"() -> (w658:i16)
                          n745 = local read "Z END"() -> (w657:i16)
                          n746 = Less?(x=w634, y=w647) -> (x < y?=w644:bool)
                          n747 = local read "Z START"() -> (w656:i16)
                          n748 = Or(x=w645, y=w644) -> (x .or. y?=w643:bool)
                          n749 = Number To Boolean Array(number=w655) -> (Boolean array=w653:bool[])
                          n750 = Boolean Array To Number(Boolean array=w653) -> (number=w654:fxp<+/-,16,16>)
                          n751 = call "LinearMove.vi"("Time"=w649, "Start"=w656, "End"=w657, "Velocity"=w654, "ExpandVelScaller"=w658) -> ("OutPosition"=w652:i16)  [unwired: 13 in, 1 out]
                          n752 = case shown="True" w640 {
                            tunnel: w638 -> [w659 w664]
                            tunnel: w637 -> [_ w663]
                            tunnel: [w659 w661] -> w636
                            tunnel: w634 -> [_ w660]
                            frame False {
                            }
                            frame True {
                              n753 = Subtract(x=w664, y=w663) -> (x-y=w662:i64)
                              n754 = Add(x=w662, y=w660) -> (x+y=w661:i64)
                            }
                          }
                        }
                      }
                      "ExtraTime 3" <- w599
                      n755 = local write "IterateHolder"(w597) -> ()
                      n756 = local write "AverageSum"(w607) -> ()
                      n757 = local write "Count Average"(w601) -> ()
                    }
                    frame 14 {
                      # "Sum of most recent 1024"
                      n758 = local read "FeedBackType"() -> (w667:u8)
                      n759 = local read "Count Average"() -> (w669:i16)
                      n760 = local read "P2AvgWhole"() -> (w668:i32)
                      n761 = case shown="1" w667 {
                        tunnel: [w680 w681 w682 w683 w684 w685] -> w666
                        frame 0, Default {
                          n762 = local read "Ext amp"() -> (w680:i16)
                        }
                        frame 1 {
                          n763 = local read "MeasuredCurrent"() -> (w681:i16)
                        }
                        frame 2 {
                          n764 = local read "MeasuredCurrent 2"() -> (w682:i16)
                        }
                        frame 3 {
                          n765 = local read "Ext Phase"() -> (w683:i16)
                        }
                        frame 4 {
                          n766 = local read "MeasuredCurrent"() -> (w684:i16)
                        }
                        frame 5 {
                          n767 = local read "MeasuredCurrent 2"() -> (w685:i16)
                        }
                      }
                      n768 = Equal?(x=w669, y=w668) -> (x = y?=w678:bool)
                      n769 = local read "ExtraTime 4"() -> (w671:fxp<+,64,64>)
                      n770 = To Long Integer(number=w666) -> (32bit integer=w665:i32)
                      n771 = local read "AverageSum"() -> (w674:i64)
                      n772 = case shown="True" w678 {
                        tunnel: w665 -> [w694 w723]
                        tunnel: w674 -> [w695 w729]
                        tunnel: [w696 w729] -> w679
                        tunnel: w669 -> [w693 w719]
                        tunnel: [w692 w719] -> w673
                        tunnel: [w691 w730] -> w677
                        tunnel: w676 -> [w689 w724]
                        tunnel: [FALSE w720] -> w675
                        tunnel: [w689 w726] -> w672
                        tunnel: w671 -> [_ w726]
                        tunnel: [w686 w718] -> w670
                        frame False {
                          n773 = local read "SampleIterator"() -> (w686:i16)
                          n774 = local read "IterateHolder"() -> (w688:i16)
                          n775 = Less?(x=w686, y=w688) -> (x < y?=w687:bool)
                          n776 = case shown="True" w687 {
                            tunnel: [w697 w704] -> w696
                            tunnel: w695 -> [w697 w703]
                            tunnel: w694 -> [_ w699]
                            tunnel: w693 -> [w698 w701]
                            tunnel: [w698 w702] -> w692
                            frame False {
                            }
                            frame True {
                              # "Count up to 1024 (start at 0) data points then start moving"
                              n777 = To Quad Integer(1:w699) -> (0:w700:i64)
                              n778 = Increment(x=w701) -> (x+1=w702:i16)
                              n779 = Add(x=w703, y=w700) -> (x+y=w704:i64)
                            }
                          }
                          n780 = local read "Applied Z"() -> (w691:i16)
                        }
                        frame True {
                          # "STOP Current Move on SetPoint"
                          n781 = local read "P2AvgMinus"() -> (w706:i32)
                          n782 = local read "Feedback_Threshold"() -> (w705:i32)
                          n783 = local read "AverageSum"() -> (w728:i64)
                          n784 = Subtract(x=w724, y=w726) -> (x-y=w727:fxp<+/-,64,65>)
                          n785 = To Quad Integer(1:w723) -> (0:w717:i64)
                          n786 = Scale By Power Of 2(n=w706, x=w728) -> (x*2^n=w713:i64)
                          n787 = To Fixed-Point(fixed-point type=w724, number=w727) -> (fixed-point=w725:fxp<+,64,64>)
                          n788 = To Quad Integer(1:w713) -> (0:w714:i64)
                          n789 = To Quad Integer(1:w705) -> (0:w709:i64)
                          n790 = Scale By Power Of 2(n=i16 15, x=w717) -> (x*2^n=w707:i64)
                          n791 = Scale By Power Of 2(n=i16 15, x=w714) -> (x*2^n=w708:i64)
                          n792 = local read "Z VEL"() -> (w733:i16)
                          n793 = local read "ExpandVelScaller Z"() -> (w736:i16)
                          n794 = Multiply(x=w713, y=w709) -> (x*y=w711:i64)
                          n795 = local read "Z END"() -> (w735:i16)
                          n796 = local read "Z START"() -> (w734:i16)
                          n797 = Number To Boolean Array(number=w733) -> (Boolean array=w731:bool[])
                          n798 = Add(x=w708, y=w711) -> (x+y=w712:i64)
                          n799 = Boolean Array To Number(Boolean array=w731) -> (number=w732:fxp<+/-,16,16>)
                          n800 = Subtract(x=w708, y=w711) -> (x-y=w710:i64)
                          n801 = Greater?(x=w707, y=w712) -> (0:w722:bool)
                          n802 = call "LinearMove.vi"("Time"=w725, "Start"=w734, "End"=w735, "Velocity"=w732, "ExpandVelScaller"=w736) -> ("OutPosition"=w730:i16)  [unwired: 13 in, 1 out]
                          n803 = Less?(x=w707, y=w710) -> (x < y?=w721:bool)
                          n804 = Or(x=w722, y=w721) -> (x .or. y?=w720:bool)
                          n805 = local read "SampleNum"() -> (w718:i16)
                        }
                      }
                      "ExtraTime 4" <- w672
                      n806 = local write "AverageSum"(w679) -> ()
                      n807 = local write "Count Average"(w673) -> ()
                      n808 = local write "IterateHolder"(w670) -> ()
                    }
                  }
                  n809 = In Range and Coerce(upper limit=32767, x=w396, lower limit=-32768) -> (coerced(x)=w395:i32)  [unwired: 1 out]
                  n810 = To Word Integer(number=w395) -> (16bit integer=w394:i16)
                  n811 = xnode "FPGA I/O Node"("Connector1/AO2"=w394) -> ()  [unwired: 1 in, 1 out]
                  n812 = local write "Applied Z"(w394) -> ()
                }
                frame #2 {
                  n813 = local read "OnlyStopLineONCE Z"() -> (w740:bool)
                  n814 = case shown="True" w740 {
                    tunnel: [w744 FALSE ("EndCurrentLine")] -> w739
                    frame False {
                      n815 = local read "EndCurrentLine"() -> (w744:bool)
                      n816 = case shown="True" w744 {
                        frame False {
                        }
                        frame True {
                          n817 = local write "OnlyStopLineONCE Z"(TRUE ("EndCurrentLine")) -> ()
                        }
                      }
                    }
                    frame True {
                    }
                  }
                  n818 = local read "External Stop"() -> (w742:bool)
                  n819 = Or(x=w737, y=w739) -> (x .or. y?=w741:bool)
                  n820 = Or(x=w742, y=w741) -> (x .or. y?=w738:bool)
                }
              }
              n821 = local write "StopMoveZ"(w357) -> ()
            }
          }
          frame True {
          }
        }
        n822 = case shown="False" w208 {
          tunnel: w206 -> [w285 _]
          frame False {
            n823 = while {
              shift-right: [w287] -> _
              shift-left: w285 -> [w290]
              stop <- w286 stop-if-true
              n824 = flat-sequence {
                tunnel: w290 -> [w292]
                tunnel: [w293] -> w291
                tunnel: w291 -> [w318]
                tunnel: [w318] -> w289
                tunnel: [w314] -> w288
                tunnel: [w349] -> w287
                tunnel: w289 -> [w349]
                tunnel: w288 -> [w343]
                tunnel: [w344] -> w286
                frame #0 {
                  n825 = local read "Internal Pause"() -> (w295:bool)
                  n826 = local read "External Pause"() -> (w296:bool)
                  n827 = Or(x=w296, y=w295) -> (x .or. y?=w294:bool)
                  n828 = case shown="True" w294 {
                    tunnel: w292 -> [w297 w300]
                    tunnel: [w297 w298] -> w293
                    frame False {
                    }
                    frame True {
                      n829 = global read "Tick Count.vi" "Tick Count"() -> (w299:u64)
                      n830 = while {
                        shift-right: [w312] -> w298
                        shift-left: w300 -> [w304]
                        shift-right: [w307] -> _
                        shift-left: w299 -> [w306]
                        stop <- w301 stop-if-true
                        n831 = local read "External Pause"() -> (w311:bool)
                        n832 = local read "Internal Pause"() -> (w309:bool)
                        n833 = global read "Tick Count.vi" "Tick Count"() -> (w307:u64)
                        n834 = local read "External Stop"() -> (w303:bool)
                        n835 = Not(x=w311) -> (.not. x?=w310:bool)
                        n836 = Not(x=w309) -> (.not. x?=w308:bool)
                        n837 = Subtract(x=w307, y=w306) -> (x-y=w305:u64)
                        n838 = And(x=w310, y=w308) -> (x .and. y?=w302:bool)
                        n839 = Add(x=w305, y=w304) -> (x+y=w312:u64)
                        n840 = Or(x=w302, y=w303) -> (x .or. y?=w301:bool)
                      }
                    }
                  }
                }
                frame #1 {
                  n841 = global read "Tick Count.vi" "Tick Count"() -> (w317:u64)
                  n842 = Subtract(x=w317, y=w318) -> (x-y=w315:u64)
                  n843 = To Fixed-Point(number=w315) -> (fixed-point=w316:fxp<+,64,64>)  [unwired: 1 in]
                  n844 = case shown="True" "Change V on Fly 2" {
                    tunnel: w316 -> [w326 _]
                    tunnel: [w325 FALSE ("Finished Move")] -> w314
                    frame False {
                      n845 = local read "V2 END"() -> (w323:i16)
                      n846 = local read "Jump V2"() -> (w324:bool)
                      n847 = case shown="True" w324 {
                        tunnel: w323 -> [w335 w336]
                        tunnel: [w334 w336] -> w320
                        tunnel: w326 -> [w333 _]
                        tunnel: [w332 TRUE ("Finished Move")] -> w325
                        frame False {
                          n848 = local read "ExpandVelScaller V2"() -> (w327:i16)
                          n849 = local read "V2 VEl"() -> (w330:i16)
                          n850 = local read "V2 START"() -> (w331:i16)
                          n851 = Number To Boolean Array(number=w330) -> (Boolean array=w329:bool[])
                          n852 = Boolean Array To Number(Boolean array=w329) -> (number=w328:fxp<+/-,16,16>)
                          n853 = call "LinearMove.vi"("Time"=w333, "Start"=w331, "End"=w335, "Velocity"=w328, "ExpandVelScaller"=w327) -> ("OutPosition"=w334:i16, "Finished Move"=w332:bool)  [unwired: 13 in]
                        }
                        frame True {
                        }
                      }
                      n854 = local read "Invert AO4 Output (V2)"() -> (w321:bool)
                      n855 = Negate(x=w320) -> (-x=w322:i16)
                      n856 = local write "Applied Voltage 2"(w320) -> ()
                      n857 = Select(t=w322, s=w321, f=w320) -> (s? t:f=w319:i16)
                      n858 = xnode "FPGA I/O Node"("Connector1/AO4"=w319) -> ()  [unwired: 1 in, 1 out]
                    }
                    frame True {
                      n859 = local read "Invert AO4 Output (V2)"() -> (w340:bool)
                      n860 = Negate(x="V2 on Fly") -> (-x=w341:i16)
                      n861 = Select(t=w341, s=w340, f="V2 on Fly") -> (s? t:f=w338:i16)
                      n862 = local write "Applied Voltage 2"("V2 on Fly") -> ()
                      n863 = xnode "FPGA I/O Node"("Connector1/AO4"=w338) -> ()  [unwired: 1 in, 1 out]
                    }
                  }
                }
                frame #2 {
                  n864 = local read "OnlyStopLineONCE V2"() -> (w345:bool)
                  n865 = case shown="False" w345 {
                    tunnel: [w350 FALSE ("EndCurrentLine")] -> w346
                    frame False {
                      n866 = local read "EndCurrentLine"() -> (w350:bool)
                      n867 = case shown="True" w350 {
                        frame False {
                        }
                        frame True {
                          n868 = local write "OnlyStopLineONCE V2"(TRUE ("EndCurrentLine")) -> ()
                        }
                      }
                    }
                    frame True {
                    }
                  }
                  n869 = Or(x=w343, y=w346) -> (x .or. y?=w348:bool)
                  n870 = local read "External Stop"() -> (w347:bool)
                  n871 = Or(x=w347, y=w348) -> (x .or. y?=w344:bool)
                }
              }
              n872 = local write "StopMoveV2"(w286) -> ()
            }
          }
          frame True {
          }
        }
      }
    }
  }
  n873 = timed-loop {
    timing: w3 -> [_]
    timing-out: [_] -> w2
    shift-right: [w1131] -> _
    shift-left: u64 0 -> [w1139]
    stop <- FALSE stop-if-true
    n874 = Split Number(x=w1139) -> (hi(x)=w1136:u32, lo(x)=w1138:u32)
    n875 = xnode "Saturation Add"("x"=w1138, "y"=u32 1) -> ("x+y"=w1132:u32, "overflow"=w1133:bool)
    n876 = Increment(x=w1136) -> (x+1=w1137:u32)
    n877 = Select(t=w1137, s=w1133, f=w1136) -> (s? t:f=w1135:u32)
    n878 = Join Numbers(hi=w1135, lo=w1132) -> ((hi.lo)=w1131:u64)
    n879 = global write "Tick Count.vi" "Tick Count"(w1131) -> ()
  }
  n880 = node-c288(w2) -> ()
  n881 = flat-sequence {
    frame #0 {
      w1218 = cluster{"LSB Weight":u32, "Offset":i32} {"LSB Weight"=0, "Offset"=0} ("Channel Calibration")
      w1219 = cluster{"LSB Weight":u32, "Offset":i32} {"LSB Weight"=0, "Offset"=0} ("Channel Calibration")
      n882 = xnode "FPGA I/O Node"("Connector1/AO3"=i16 0 ("Connector1/AO7")) -> ("FPGA I/O Out"=w1181:refnum<k21>)  [unwired: 1 in]
      n883 = xnode "FPGA I/O Node"("Connector1/AO1"=i16 16383 ("Connector1/AO7")) -> ("FPGA I/O Out"=w1179:refnum<k21>)  [unwired: 1 in]
      n884 = xnode "FPGA I/O Node"("Connector1/AO2"=i16 16383 ("Connector1/AO7")) -> ("FPGA I/O Out"=w1180:refnum<k21>)  [unwired: 1 in]
      n885 = xnode "FPGA I/O Node"("Connector1/AO0"=i16 16383 ("Connector1/AO7")) -> ("FPGA I/O Out"=w1178:refnum<k21>)  [unwired: 1 in]
      n886 = xnode "FPGA I/O Node"() -> ("FPGA I/O Out"=w1201:refnum<k21>)  [unwired: 1 in, 1 out]
      n887 = xnode "FPGA I/O Node"() -> ("FPGA I/O Out"=w1202:refnum<k21>)  [unwired: 1 in, 1 out]
      n888 = xnode "FPGA I/O Node"() -> ("FPGA I/O Out"=w1203:refnum<k21>)  [unwired: 1 in, 1 out]
      n889 = xnode "FPGA I/O Node"() -> ("FPGA I/O Out"=w1200:refnum<k21>)  [unwired: 1 in, 1 out]
      n890 = xnode "FPGA I/O Node"("Connector1/AO7"=i16 0) -> ("FPGA I/O Out"=w1185:refnum<k21>)  [unwired: 1 in]
      n891 = xnode "FPGA I/O Node"("Connector1/AO6"=i16 0 ("Connector1/AO7")) -> ("FPGA I/O Out"=w1184:refnum<k21>)  [unwired: 1 in]
      n892 = xnode "FPGA I/O Node"("Connector1/AO5"=i16 0 ("Connector1/AO7")) -> ("FPGA I/O Out"=w1183:refnum<k21>)  [unwired: 1 in]
      n893 = xnode "FPGA I/O Node"("Connector1/AO4"=i16 0 ("Connector1/AO7")) -> ("FPGA I/O Out"=w1182:refnum<k21>)  [unwired: 1 in]
      n894 = xnode "FPGA I/O Node"() -> ("FPGA I/O Out"=w1204:refnum<k21>)  [unwired: 1 in, 1 out]
      n895 = xnode "FPGA I/O Node"() -> ("FPGA I/O Out"=w1205:refnum<k21>)  [unwired: 1 in, 1 out]
      n896 = xnode "FPGA I/O Node"() -> ("FPGA I/O Out"=w1206:refnum<k21>)  [unwired: 1 in, 1 out]
      n897 = xnode "FPGA I/O Node"() -> ("FPGA I/O Out"=w1209:refnum<k21>)  [unwired: 1 in, 1 out]
      n898 = xnode "FPGA I/O Property Node"("FPGA I/O In"=w1179) -> ("LSB Weight"=w1165:u32, "Offset"=w1164:i32)  [unwired: 1 out]
      n899 = xnode "FPGA I/O Property Node"("FPGA I/O In"=w1180) -> ("LSB Weight"=w1167:u32, "Offset"=w1166:i32)  [unwired: 1 out]
      n900 = xnode "FPGA I/O Property Node"("FPGA I/O In"=w1178) -> ("LSB Weight"=w1163:u32, "Offset"=w1162:i32)  [unwired: 1 out]
      n901 = xnode "FPGA I/O Property Node"("FPGA I/O In"=w1201) -> ("LSB Weight (+/- 10 V range)"=w1189:u32, "Offset (+/- 10 V range)"=w1188:i32)  [unwired: 1 out]
      n902 = xnode "FPGA I/O Property Node"("FPGA I/O In"=w1202) -> ("LSB Weight (+/- 10 V range)"=w1191:u32, "Offset (+/- 10 V range)"=w1190:i32)  [unwired: 1 out]
      n903 = xnode "FPGA I/O Property Node"("FPGA I/O In"=w1203) -> ("LSB Weight (+/- 10 V range)"=w1193:u32, "Offset (+/- 10 V range)"=w1192:i32)  [unwired: 1 out]
      n904 = xnode "FPGA I/O Property Node"("FPGA I/O In"=w1181) -> ("LSB Weight"=w1169:u32, "Offset"=w1168:i32)  [unwired: 1 out]
      n905 = xnode "FPGA I/O Property Node"("FPGA I/O In"=w1200) -> ("LSB Weight (+/- 10 V range)"=w1187:u32, "Offset (+/- 10 V range)"=w1186:i32)  [unwired: 1 out]
      n906 = xnode "FPGA I/O Property Node"("FPGA I/O In"=w1185) -> ("LSB Weight"=w1177:u32, "Offset"=w1176:i32)  [unwired: 1 out]
      n907 = xnode "FPGA I/O Property Node"("FPGA I/O In"=w1184) -> ("LSB Weight"=w1175:u32, "Offset"=w1174:i32)  [unwired: 1 out]
      n908 = xnode "FPGA I/O Property Node"("FPGA I/O In"=w1183) -> ("LSB Weight"=w1173:u32, "Offset"=w1172:i32)  [unwired: 1 out]
      n909 = xnode "FPGA I/O Property Node"("FPGA I/O In"=w1182) -> ("LSB Weight"=w1171:u32, "Offset"=w1170:i32)  [unwired: 1 out]
      n910 = xnode "FPGA I/O Property Node"("FPGA I/O In"=w1204) -> ("LSB Weight (+/- 10 V range)"=w1195:u32, "Offset (+/- 10 V range)"=w1194:i32)  [unwired: 1 out]
      n911 = xnode "FPGA I/O Property Node"("FPGA I/O In"=w1205) -> ("LSB Weight (+/- 10 V range)"=w1197:u32, "Offset (+/- 10 V range)"=w1196:i32)  [unwired: 1 out]
      n912 = xnode "FPGA I/O Property Node"("FPGA I/O In"=w1206) -> ("LSB Weight (+/- 10 V range)"=w1199:u32, "Offset (+/- 10 V range)"=w1198:i32)  [unwired: 1 out]
      n913 = xnode "FPGA I/O Property Node"("FPGA I/O In"=w1209) -> ("LSB Weight (+/- 10 V range)"=w1208:u32, "Offset (+/- 10 V range)"=w1207:i32)  [unwired: 1 out]
      n914 = Bundle(cluster=w1219, "LSB Weight"=w1187, "Offset"=w1186) -> (→"CalCoefAi7":cluster{"LSB Weight":u32, "Offset":i32})
      n915 = Bundle(cluster=w1219, "LSB Weight"=w1191, "Offset"=w1190) -> (→"CalCoefAi5":cluster{"LSB Weight":u32, "Offset":i32})
      n916 = Bundle(cluster=w1219, "LSB Weight"=w1195, "Offset"=w1194) -> (→"CalCoefAi3":cluster{"LSB Weight":u32, "Offset":i32})
      n917 = Bundle(cluster=w1219, "LSB Weight"=w1189, "Offset"=w1188) -> (→"CalCoefAi6":cluster{"LSB Weight":u32, "Offset":i32})
      n918 = Bundle(cluster=w1219, "LSB Weight"=w1193, "Offset"=w1192) -> (→"CalCoefAi4":cluster{"LSB Weight":u32, "Offset":i32})
      n919 = Bundle(cluster=w1219, "LSB Weight"=w1197, "Offset"=w1196) -> (→"CalCoefAi2":cluster{"LSB Weight":u32, "Offset":i32})
      n920 = Bundle(cluster=w1219, "LSB Weight"=w1199, "Offset"=w1198) -> (→"CalCoefAi1":cluster{"LSB Weight":u32, "Offset":i32})
      n921 = Bundle(cluster=w1219, "LSB Weight"=w1208, "Offset"=w1207) -> (→"CalCoefAi0":cluster{"LSB Weight":u32, "Offset":i32})
      n922 = Bundle(cluster=w1218, "LSB Weight"=w1177, "Offset"=w1176) -> (→"CalCoefAo7":cluster{"LSB Weight":u32, "Offset":i32})
      n923 = Bundle(cluster=w1218, "LSB Weight"=w1173, "Offset"=w1172) -> (→"CalCoefAo5":cluster{"LSB Weight":u32, "Offset":i32})
      n924 = Bundle(cluster=w1218, "LSB Weight"=w1169, "Offset"=w1168) -> (→"CalCoefAo3":cluster{"LSB Weight":u32, "Offset":i32})
      n925 = Bundle(cluster=w1218, "LSB Weight"=w1175, "Offset"=w1174) -> (→"CalCoefAo6":cluster{"LSB Weight":u32, "Offset":i32})
      n926 = Bundle(cluster=w1218, "LSB Weight"=w1171, "Offset"=w1170) -> (→"CalCoefAo4":cluster{"LSB Weight":u32, "Offset":i32})
      n927 = Bundle(cluster=w1218, "LSB Weight"=w1167, "Offset"=w1166) -> (→"CalCoefAo2":cluster{"LSB Weight":u32, "Offset":i32})
      n928 = Bundle(cluster=w1218, "LSB Weight"=w1165, "Offset"=w1164) -> (→"CalCoefAo1":cluster{"LSB Weight":u32, "Offset":i32})
      n929 = Bundle(cluster=w1218, "LSB Weight"=w1163, "Offset"=w1162) -> (→"CalCoefAo0":cluster{"LSB Weight":u32, "Offset":i32})
    }
    frame #1 {
      "CalConstants Ready" <- TRUE ("CalConstantsReady")
    }
  }
